vi "TestSequenceSubVI.vi"(0 "GuiRef":T2={"StringOut"=refnum, "AbortOnFail"=refnum, "SN"=refnum, "SN_Length"=refnum, "TestResult"=refnum, "CycleTime"=refnum, "ErrorCode"=refnum, "UUTStatus"=refnum, "DataBaseEnable?"=refnum, "DUTModel"=refnum, "FixtureID"=refnum, "OperatorID"=refnum, "SNReady"=refnum, "StopSlot"=refnum, "NextStep"=refnum, "PassYeild"=refnum, "Failed"=refnum, "Passed"=refnum, "Tested"=refnum, "TestItemsCtl"={"StepName"="", "TestEnable"=FALSE, "LoopCount"=0, "StopOnFail"=FALSE, "Index"=0, "TestName"="", "通道"="", "参数"="", "TimeStart"=0}, "ProcessBar"=refnum, "Slot"=enum."Slot1", "Row"=3, "States"=refnum, "TestMode"=refnum, "循环次数-DUT"=refnum, "波形图"=refnum, "产品型号"=refnum, "子面板"=refnum, "测试失败项目"=refnum, "测试结果"=refnum, "DUT"=refnum, "Starttime"=refnum, "SlotReady"=refnum, "版本信息"=refnum}, 7 "MSComm":refnum<k7>, 11 "error in":errorcluster, 14 "semaphore":T1 caption="信号量") -> (15 "error out":errorcluster)   [LabVIEW 2013]
uses:
  SystemCode/SysControl/Reference.ctl
  SystemCode/SysControl/TestItemsCTL.ctl
  SystemCode/SysControl/Slot.ctl
  SourceCode/CCID info.ctl
  <vilib>/measure/matone.llb/Extract Single Tone Information 1 Chan.vi
  SourceCode/GlobalValue.vi
  <vilib>/measure/madcrms.llb/Basic Averaged DC-RMS for 1 Chan.vi
  <vilib>/measure/matone.llb/SINAD Analyzer 1 Chan.vi
  <vilib>/addons/Sound and Vibration/svt_Distortion/SVT THD+N (Time) (1 Ch).vi
  <vilib>/ErrorRing/Error Ring.xnode
  <vilib>/measure/NI_MAPro.lvlib
  <vilib>/addons/Sound and Vibration/svt_Distortion/SoundVib_Distortion.lvlib
panel:
  out "错误输出":errorcluster
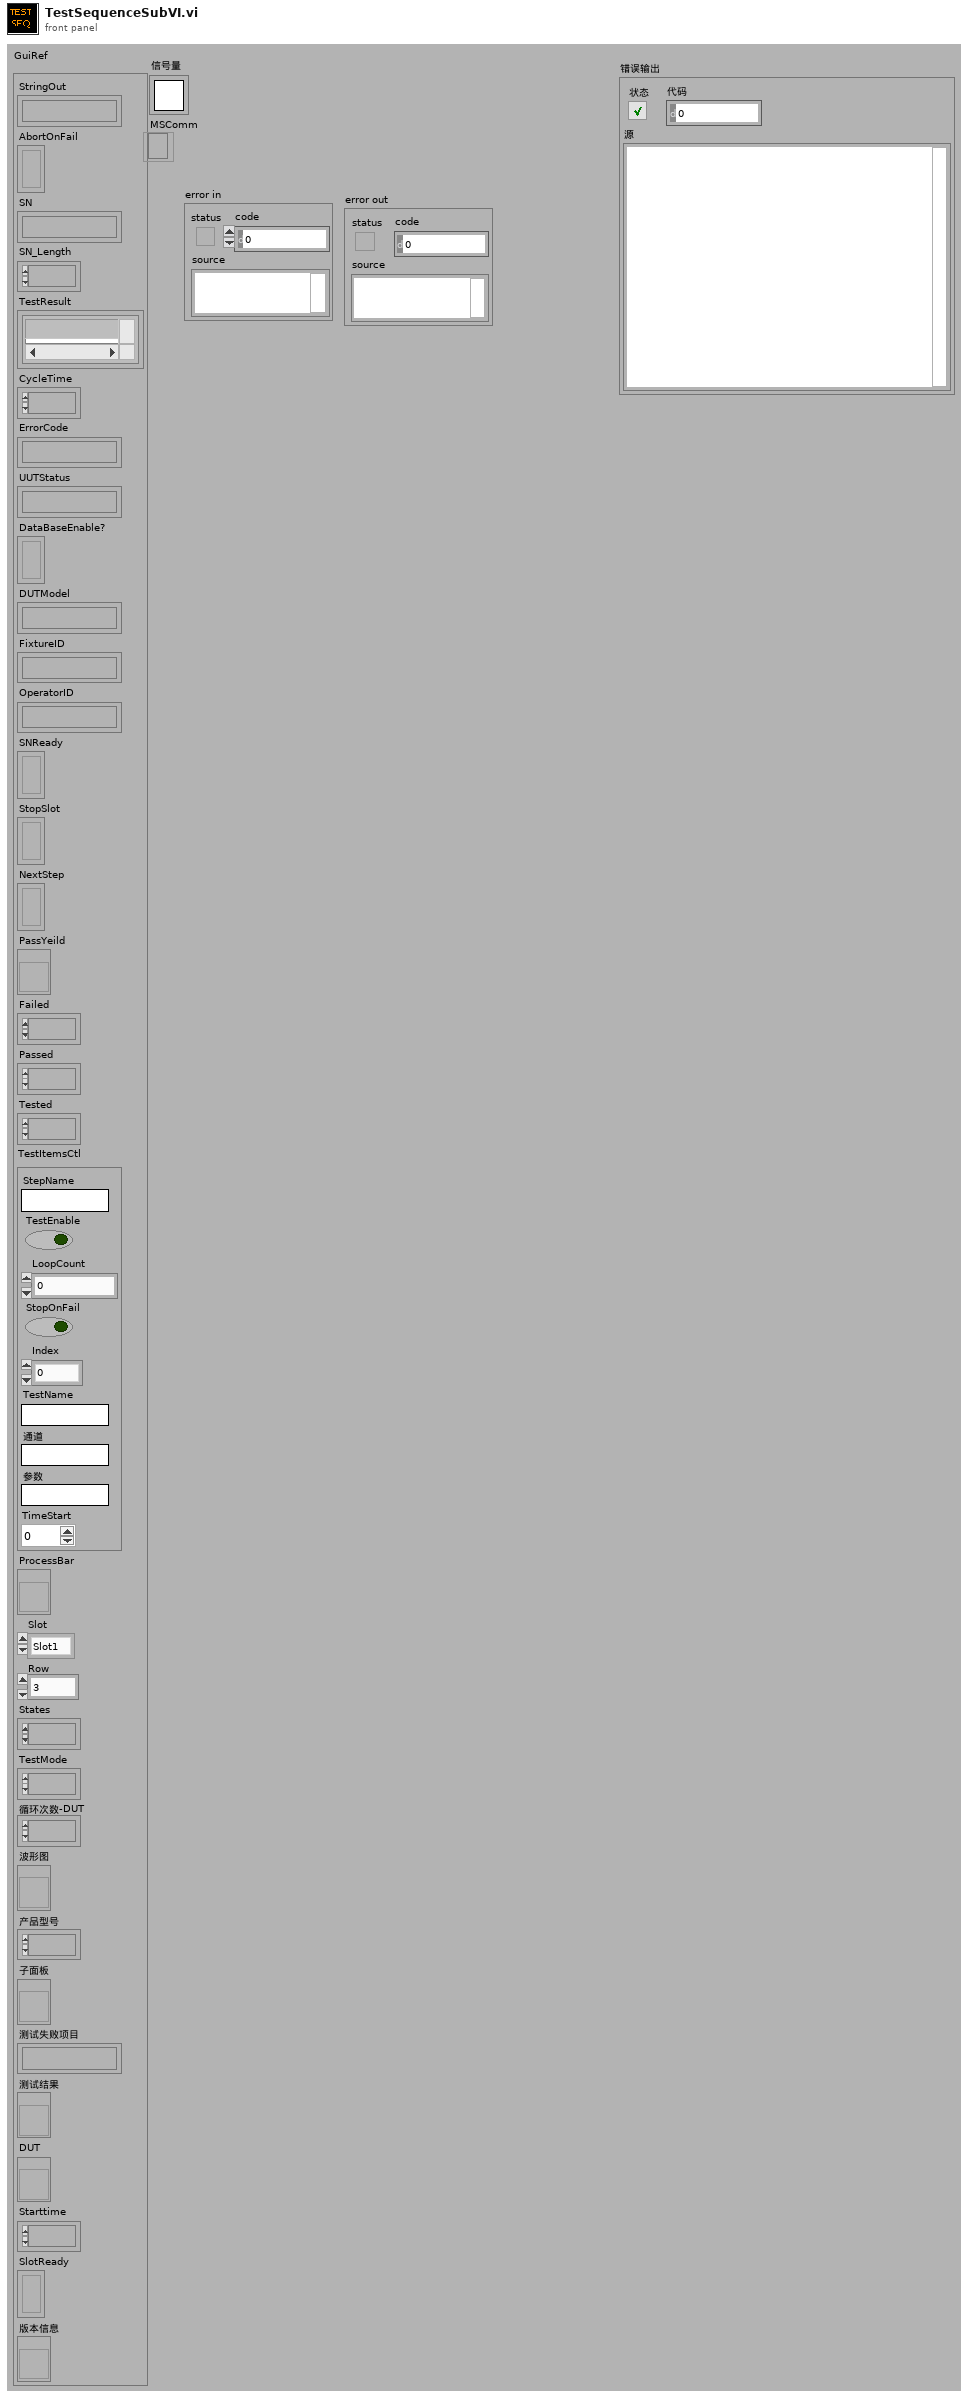
[diagram p1: front panel]
types:
  T1 = typedef "Semaphore RefNum" = refnum<k1>
  T2 = typedef "Reference.ctl" = cluster{"StringOut":refnum<vi>, "AbortOnFail":refnum<vi>, "SN":refnum<vi>, "SN_Length":refnum<vi>, "TestResult":refnum<vi>, "CycleTime":refnum<vi>, "ErrorCode":refnum<vi>, "UUTStatus":refnum<vi>, "DataBaseEnable?":refnum<vi>, "DUTModel":refnum<vi>, "FixtureID":refnum<vi>, "OperatorID":refnum<vi>, "SNReady":refnum<vi>, "StopSlot":refnum<vi>, "NextStep":refnum<vi>, "PassYeild":refnum<vi>, "Failed":refnum<vi>, "Passed":refnum<vi>, "Tested":refnum<vi>, "TestItemsCtl":T3, "ProcessBar":refnum<vi>, "Slot":T4, "Row":u32, "States":refnum<vi>, "TestMode":refnum<vi>, "循环次数-DUT":refnum<vi>, "波形图":refnum<vi>, "产品型号":refnum<vi>, "子面板":refnum<vi>, "测试失败项目":refnum<vi>, "测试结果":refnum<vi>, "DUT":refnum<vi>, "Starttime":refnum<vi>, "SlotReady":refnum<vi>, "版本信息":refnum<vi>}
  T3 = typedef "TestItemsCTL.ctl" = cluster{"StepName":string, "TestEnable":bool, "LoopCount":i32, "StopOnFail":bool, "Index":u32, "TestName":string, "通道":string, "参数":string, "TimeStart":u32}
  T4 = typedef "Slot.ctl" = enum16{"Slot1", "Slot2", "Slot3", "Slot4"}
  T5 = cluster{"THD+N units":enum16{"dB", "linear ratio", "%"}, "detected fundamental amplitude units":enum16{"EU rms", "EU peak", "EU peak-peak"}}
  T6 = typedef "CCID info.ctl" = enum16{"Fw Ver", "HW Ver", "CCID", "WiFiName", "DevID"}
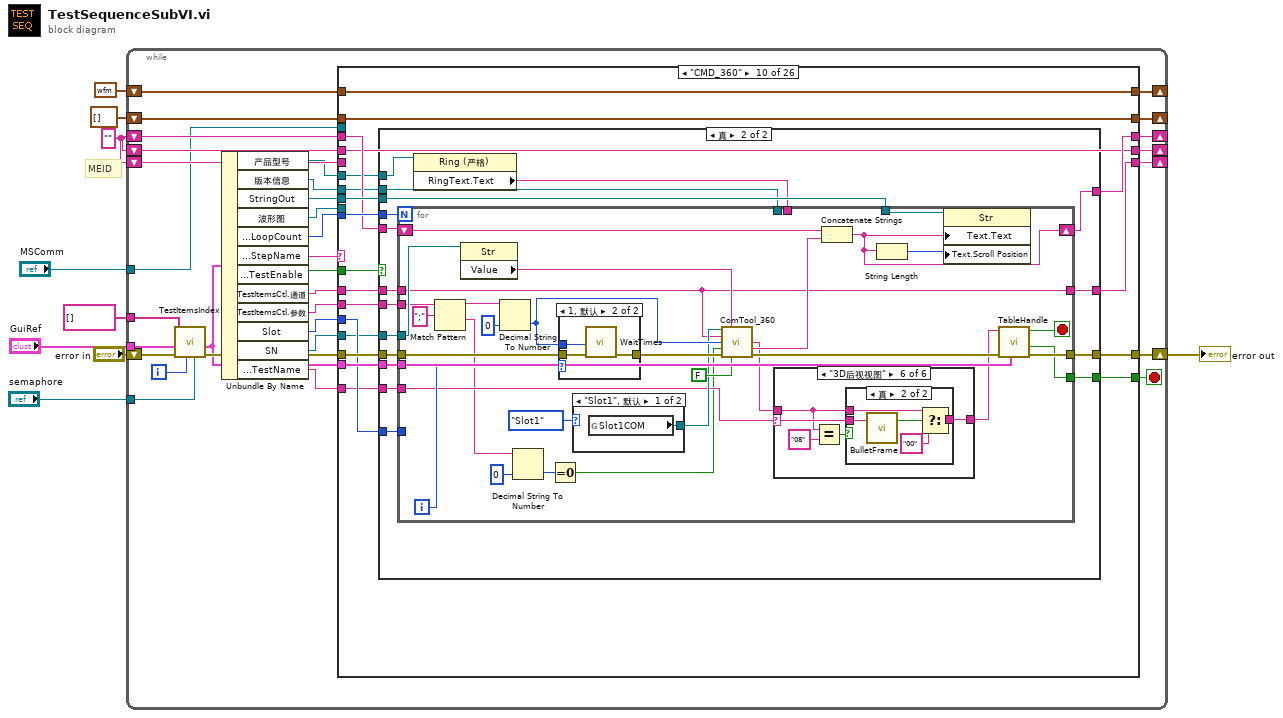
[diagram p0: block diagram]
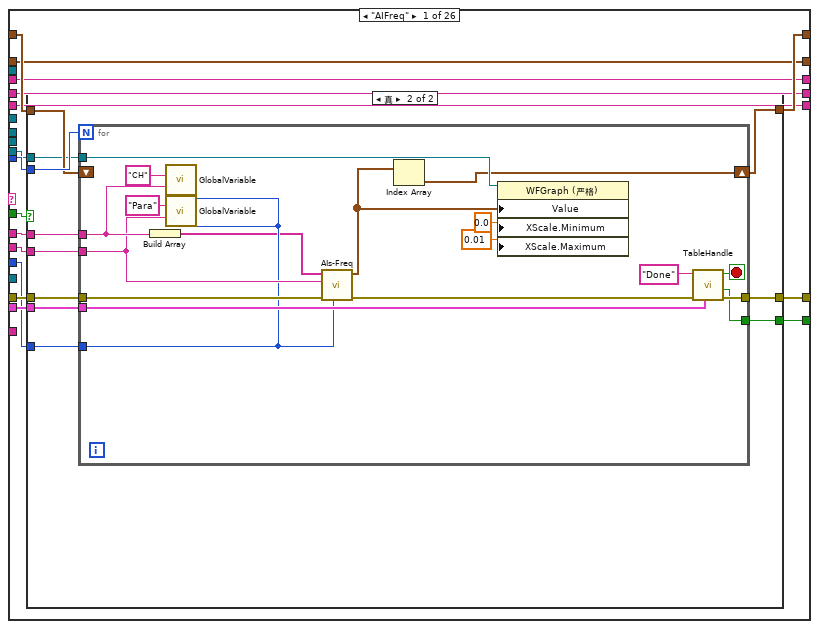
[diagram p2: hidden frame]
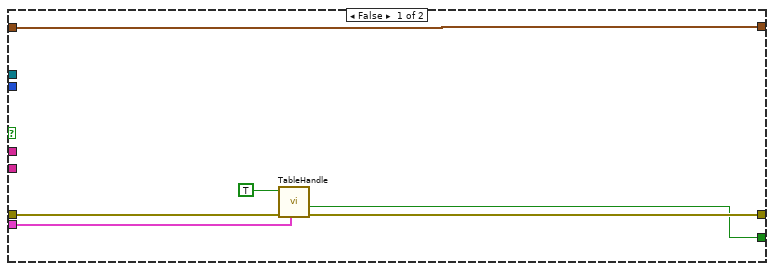
[diagram p3: hidden frame]
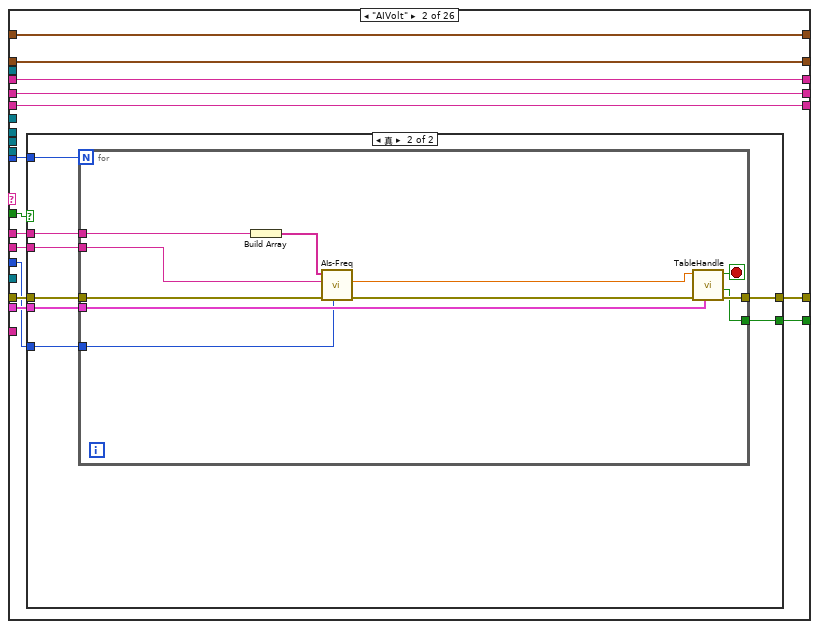
[diagram p4: hidden frame]
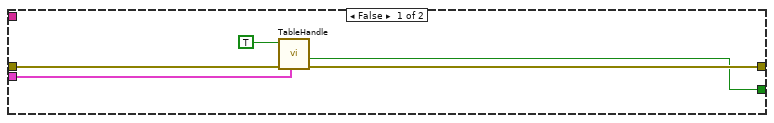
[diagram p5: hidden frame]
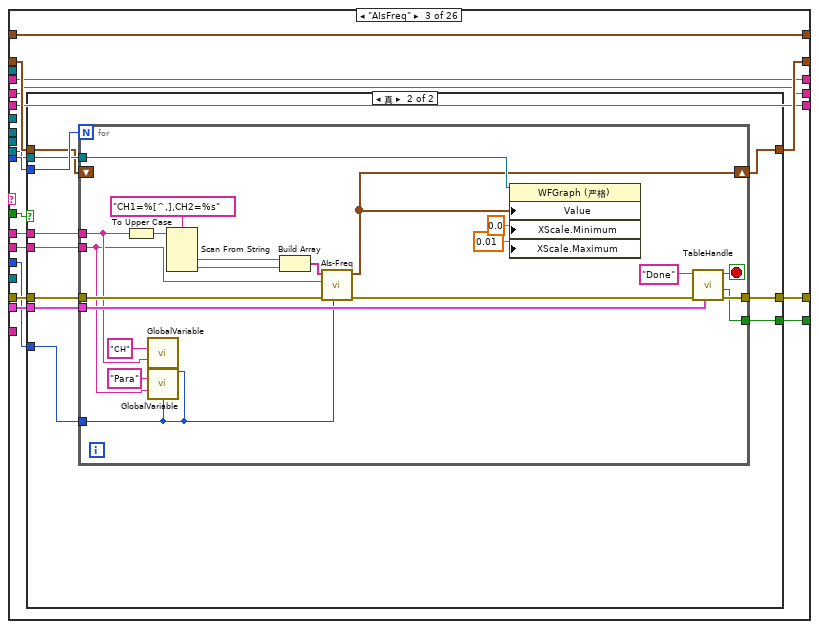
[diagram p6: hidden frame]
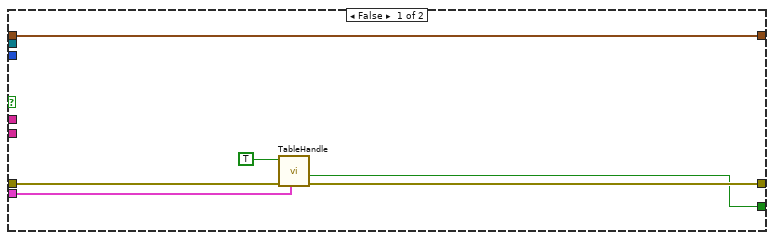
[diagram p7: hidden frame]
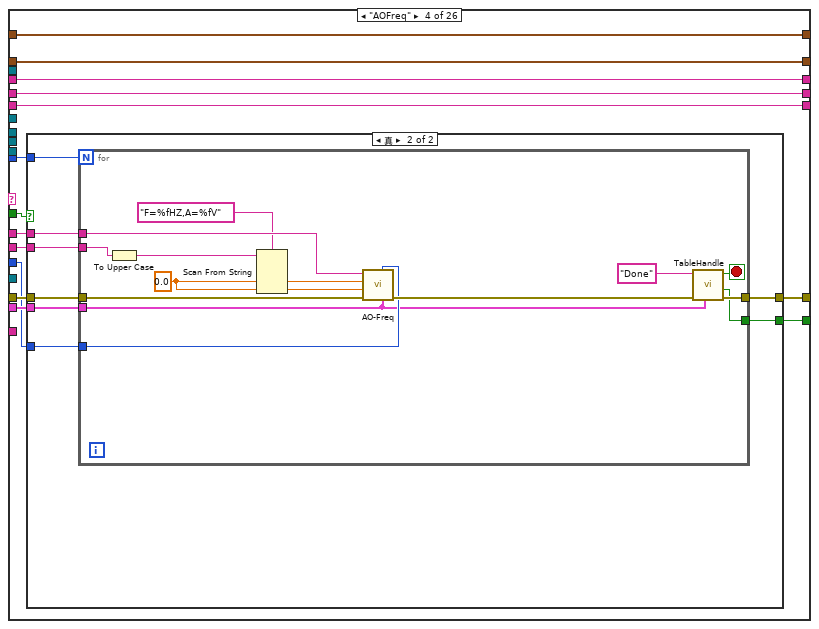
[diagram p8: hidden frame]
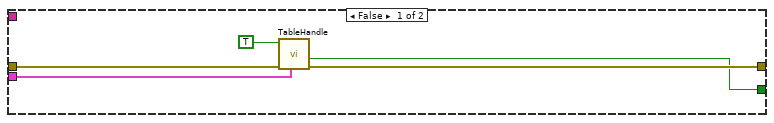
[diagram p9: hidden frame]
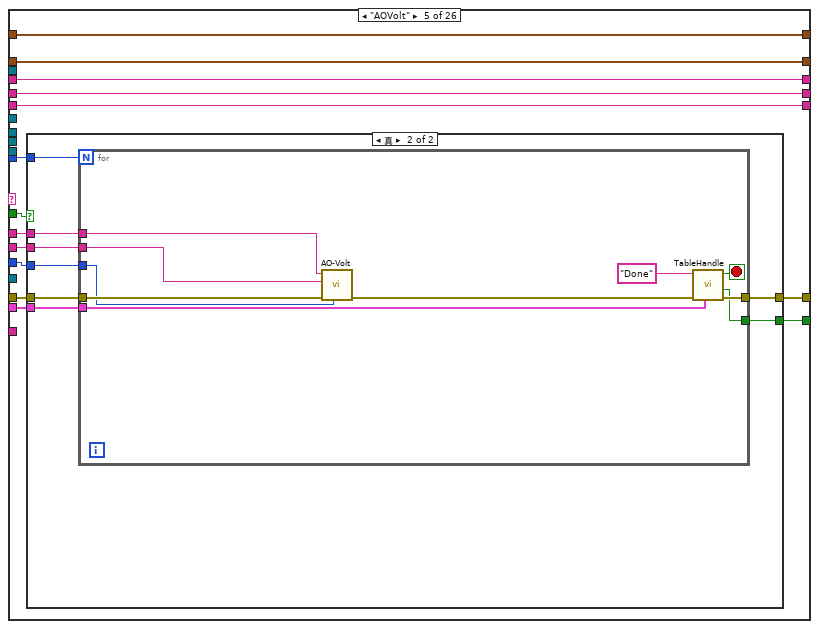
[diagram p10: hidden frame]
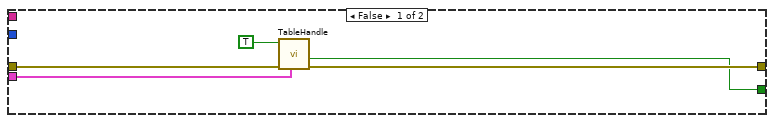
[diagram p11: hidden frame]
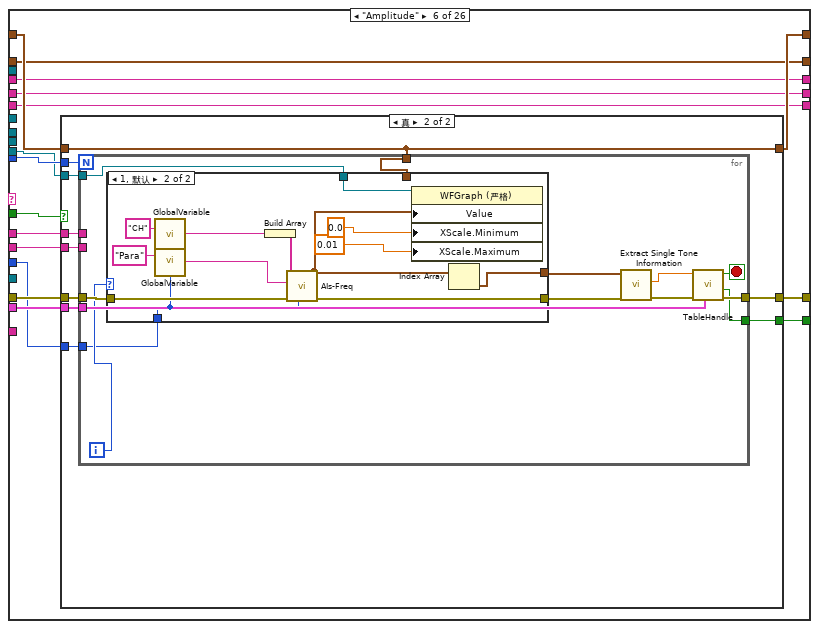
[diagram p12: hidden frame]
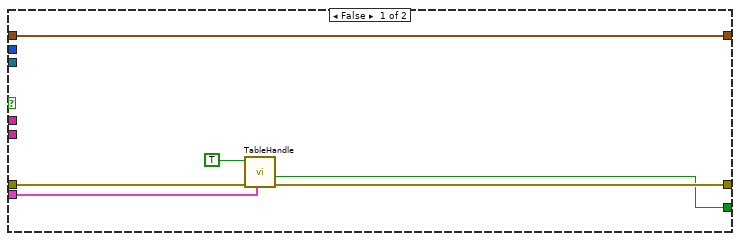
[diagram p13: hidden frame]
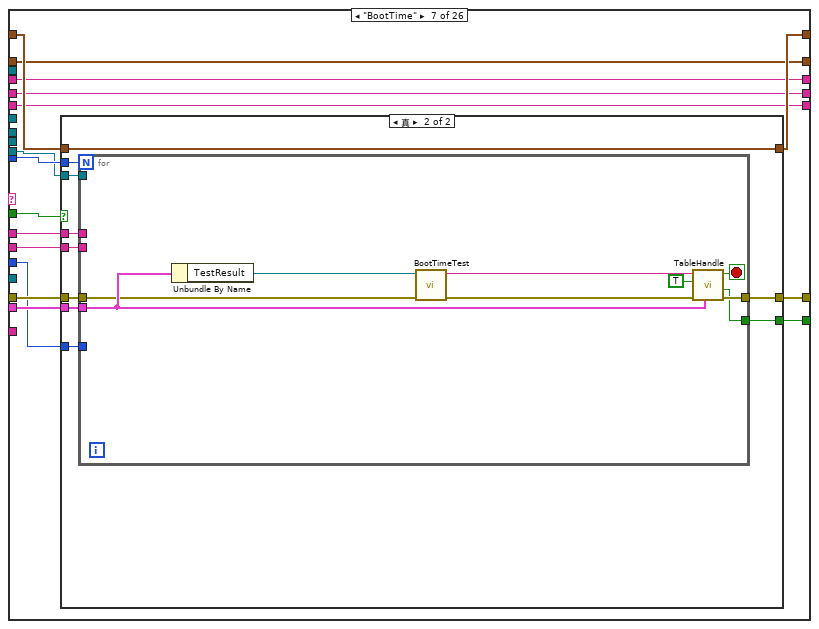
[diagram p15: hidden frame]
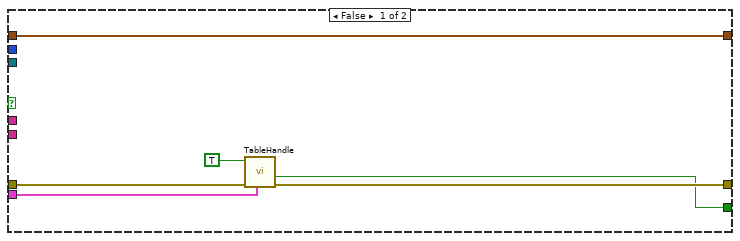
[diagram p16: hidden frame]
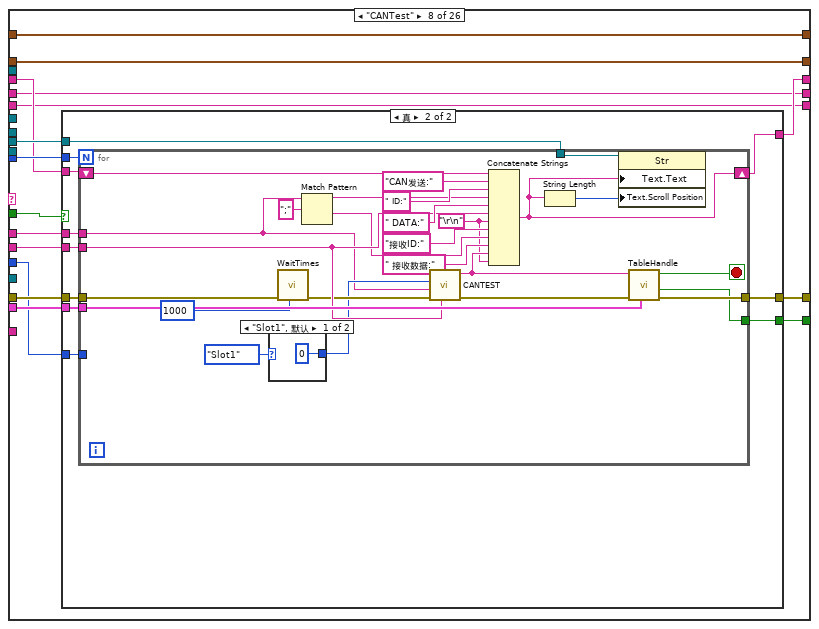
[diagram p17: hidden frame]
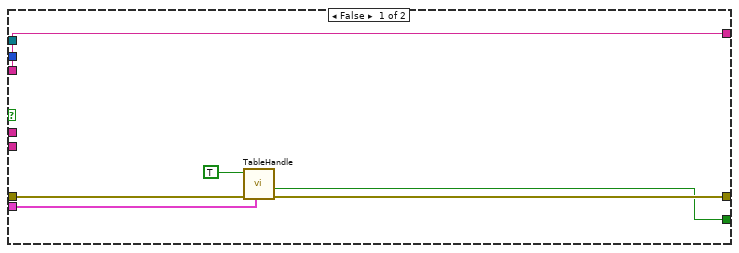
[diagram p18: hidden frame]
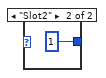
[diagram p19: hidden frame]
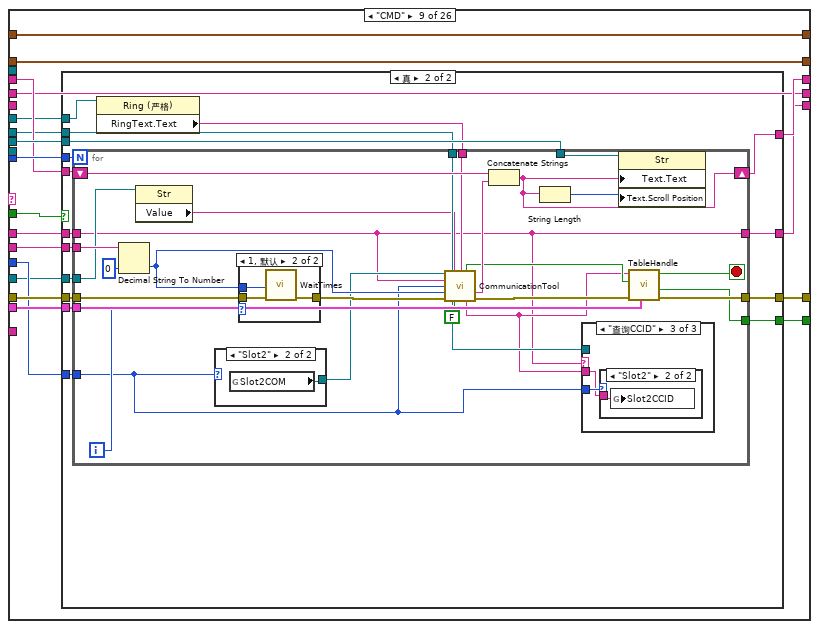
[diagram p20: hidden frame]
diagram:
  w2 = "" ("CMD")
  # "MEID"
  n1 = while {
    shift-right: [w37] -> w9
    shift-left: "error in" -> [w41]
    tunnel: "GuiRef" -> [w35]
    shift-right: [w29] -> _
    shift-left: waveform(dbl) {"t0"=timestamp(0 s since 1904-01-01), "dt"=1.0, "Y"=[]} ("Raw Data 3") -> [w28]
    shift-right: [w27] -> _
    shift-left: waveform(dbl)[] [] ("波形图") -> [w26]
    shift-right: [w23] -> _
    shift-left: w2 -> [w22]
    tunnel: string[] [] ("Fail项目") -> [w21]
    tunnel: "semaphore" -> [w19]
    shift-right: [w18] -> _
    shift-left: w2 -> [w17]
    shift-right: [w15] -> _
    shift-left: w2 -> [w16]
    tunnel: "MSComm" -> [w11]
    i -> [w20]
    stop <- w36 stop-if-true
    n2 = call "TestItemsIndex.vi"("semaphore"=w19, "TestItemIndexIn"=w20, "ErrorIn(NoError)"=w41, "GuiRef"=w35, "Fail项目"=w21) -> ("ErrorOut"=w40:errorcluster, "GuiRefOut"=w34:T2)  [unwired: 5 out]
    n3 = Unbundle By Name(w34) -> ("产品型号"=w12:refnum<vi>, "版本信息"=w14:refnum<vi>, "StringOut"=w24:refnum<vi>, "波形图"=w25:refnum<vi>, "TestItemsCtl.LoopCount"=w30:i32, "TestItemsCtl.StepName"=w39:string, "TestItemsCtl.TestEnable"=w38:bool, "TestItemsCtl.通道"=w31:string, "TestItemsCtl.参数"=w32:string, "Slot"=w33:T4, "SN"=w13:refnum<vi>, "TestItemsCtl.TestName"=w10:string)
    n4 = case shown="\"CMD_360\"" w39 {
      selector: w39 -> [_ _ _ _ _ _ _ _ _ _ _ _ _ _ _ _ _ _ _ _ _ _ _ _ _ w1271]
      tunnel: [w55 w104 w144 w196 w238 w277 w337 w378 w442 w522 w654 w694 w730 w767 w807 w844 w907 w967 w1035 w1063 w1117 w1131 w1187 w1223 w1236 w1275] -> w37
      tunnel: w40 -> [w56 w105 w145 w197 w239 w278 w338 w379 w443 w523 w655 w695 w731 w768 w808 w845 w908 w968 w1036 w1067 w1117 w1132 _ w1223 w1237 _]
      tunnel: w34 -> [w57 w106 w146 w198 w240 w279 w339 w380 w444 w524 w656 w696 w732 w769 w809 w846 w909 w969 w1037 w1066 _ w1133 w1182 _ w1238 _]
      tunnel: w38 -> [w54 w103 w143 w195 w237 w276 w336 w377 w441 w521 w653 w693 w729 w766 w806 w843 w906 w966 w1034 w1061 _ w1130 _ _ w1235 _]
      tunnel: [w53 w102 w142 w194 w236 w275 w335 w376 w440 w520 w652 w692 w728 w765 w805 w842 w905 w965 w1033 w1064 TRUE ("StopOnFail?") w1129 w1186 FALSE ("StopOnFail?") w1234 TRUE ("StopOnFail?")] -> w36
      tunnel: w33 -> [w52 w101 w141 w193 w235 w274 w334 w375 w439 w519 w651 w691 w727 w764 w804 w841 w904 w964 w1032 w1065 _ w1128 w1190 _ w1233 w1266]
      tunnel: w32 -> [w50 w99 w139 w191 w233 w272 w332 w373 w437 w517 w649 w689 w725 w762 w802 w839 w902 w962 w1030 w1068 _ w1126 _ _ w1231 _]
      tunnel: w31 -> [w51 w100 w140 w192 w234 w273 w333 w374 w438 w518 w650 w690 w726 w763 w803 w840 w903 w963 w1031 w1069 _ w1127 w1191 _ w1232 _]
      tunnel: w30 -> [w49 w98 w138 w190 w232 w271 w331 w372 w436 w516 w648 w688 w724 w761 w801 w838 w901 w961 w1029 w1070 _ w1125 _ _ w1230 _]
      tunnel: [w48 w97 w137 w189 w231 w269 w329 w371 w435 w515 w646 w687 w723 w760 w799 w837 w899 w959 w1028 w1062 w1115 w1123 w1184 w1221 w1228 w1274] -> w29
      tunnel: w28 -> [w47 w97 w137 w189 w231 w270 w330 w371 w435 w515 w647 w687 w723 w760 w800 w837 w900 w960 w1028 w1062 w1115 w1124 w1184 w1221 w1229 w1274]
      tunnel: [w46 w96 w136 w188 w230 w268 w328 w370 w434 w514 w645 w686 w722 w759 w798 w836 w898 w958 w1027 w1074 w1114 w1122 w1195 w1220 w1227 w1273] -> w27
      tunnel: w26 -> [w46 w96 w135 w188 w230 w268 w328 w370 w434 w514 w645 w686 w722 w759 w798 w836 w898 w958 w1027 w1074 w1114 w1122 w1195 w1220 w1227 w1273]
      tunnel: w25 -> [w45 _ w134 _ _ w266 w326 _ _ _ _ _ _ _ _ _ w896 w956 _ _ _ w1120 _ _ _ _]
      tunnel: w24 -> [_ _ _ _ _ _ _ w369 w433 w513 _ _ _ _ _ _ _ _ _ _ _ _ _ _ _ _]
      tunnel: [w44 w95 w133 w187 w229 w267 w327 w368 w432 w512 w644 w685 w721 w758 w797 w835 w897 w957 w1026 w1073 w1113 w1121 w1194 w1219 w1226 w1268] -> w23
      tunnel: w22 -> [w44 w95 w133 w187 w229 w267 w327 w367 w431 w511 w644 w685 w721 w758 w797 w835 w897 w957 w1026 w1073 w1113 w1121 w1194 w1219 w1226 w1268]
      tunnel: [w43 w94 w132 w186 w228 w265 w325 w366 w430 w510 w643 w684 w720 w757 w796 w834 w895 w955 w1025 w1072 w1112 w1119 w1193 w1218 w1225 w1264] -> w18
      tunnel: w17 -> [w43 w94 w132 w186 w228 w265 w325 w366 w430 w510 w643 w684 w720 w757 w796 w834 w895 w955 w1025 w1072 w1112 w1119 w1193 w1218 w1225 w1264]
      tunnel: w16 -> [w42 w93 w131 w185 w227 w264 w324 w365 _ _ w642 w683 w719 w756 w795 w833 w894 w954 w1024 w1071 w1111 w1118 w1192 w1217 w1224 w1263]
      tunnel: [w42 w93 w131 w185 w227 w264 w324 w365 w429 w509 w642 w683 w719 w756 w795 w833 w894 w954 w1024 w1071 w1111 w1118 w1192 w1217 w1224 w1263] -> w15
      tunnel: w14 -> [_ _ _ _ _ _ _ _ w428 w508 _ _ _ _ _ _ _ _ _ _ _ _ _ _ _ _]
      tunnel: w13 -> [_ _ _ _ _ _ _ _ w427 w507 w641 _ _ _ _ _ _ _ _ _ _ _ w1188 _ _ _]
      tunnel: w12 -> [_ _ _ _ _ _ _ _ w426 w506 _ _ _ _ _ _ _ _ _ _ _ _ w1189 _ _ _]
      tunnel: w11 -> [_ _ _ _ _ _ _ _ _ _ _ _ _ _ _ _ _ _ _ _ _ _ _ _ _ _]
      tunnel: w10 -> [_ _ _ _ _ _ _ _ _ w505 _ _ _ _ _ _ _ _ _ _ _ _ _ _ _ _]
      frame "AIFreq" {
        n5 = case shown="真" w54 {
          tunnel: w57 -> [w61 w72]
          tunnel: w56 -> [w62 w74]
          tunnel: [w63 w73] -> w55
          tunnel: [w60 w71] -> w53
          tunnel: w52 -> [_ w70]
          tunnel: w51 -> [_ w69]
          tunnel: w50 -> [_ w68]
          tunnel: w49 -> [_ w67]
          tunnel: [w58 w66] -> w48
          tunnel: w47 -> [w58 w65]
          tunnel: w45 -> [_ w64]
          frame False {
            n6 = call "TableHandle.vi"("All"=w61, "error in (no error)"=w62, "DataIn"=TRUE) -> ("error out"=w63:errorcluster, "Stop?"=w60:bool)  [unwired: 3 in, 4 out]
          }
          frame True {
            n7 = for "For循环" {
              N: w67 -> [_]
              tunnel: w74 -> [w88]
              tunnel: [w92] -> w73
              tunnel: w72 -> [w89]
              tunnel: [w90] -> w71
              tunnel: w70 -> [w77]
              tunnel: w68 -> [w78]
              tunnel: w69 -> [w80]
              shift-right: [w82] -> w66
              shift-left: w65 -> [_]
              tunnel: w64 -> [w84]
              stop <- w91 stop-if-true
              n8 = Build Array(w80) -> (w76:string[])
              n9 = call "GlobalVariable.vi"("Name"="CH", "ValueIn"=w80, "Slot"=w77) -> ()  [unwired: 9 in, 4 out]
              n10 = call "GlobalVariable.vi"("Name"="Para", "ValueIn"=w78, "Slot"=w77) -> ()  [unwired: 9 in, 4 out]
              n11 = call "AIs-Freq.vi"("Slot"=w77, "error in"=w88, "Mode"=w78, "CHs"=w76) -> ("error out"=w87:errorcluster, "波形图"=w75:waveform(dbl)[])  [unwired: 5 in, 1 out]
              n12 = Index Array(array=w75) -> (element=w82:waveform(dbl))  [unwired: 1 in]
              n13 = property class="WFGraph (严格)"(reference=w84, "Value"=w75, "XScale.Minimum"=0.0 ("X标尺.范围:最小值"), "XScale.Maximum"=0.01 ("X标尺.范围:最大值")) -> ()  [unwired: 1 in, 2 out]
              n14 = call "TableHandle.vi"("All"=w89, "error in (no error)"=w87, "DataIn"="Done") -> ("error out"=w92:errorcluster, "Stop?"=w90:bool, "StopForLoop"=w91:bool)  [unwired: 4 in, 2 out]
            }
          }
        }
      }
      frame "AIVolt" {
        n15 = case shown="真" w103 {
          tunnel: w106 -> [w109 w117]
          tunnel: w105 -> [w110 w119]
          tunnel: [w111 w118] -> w104
          tunnel: [w108 w116] -> w102
          tunnel: w101 -> [_ w115]
          tunnel: w100 -> [_ w114]
          tunnel: w99 -> [_ w113]
          tunnel: w98 -> [_ w112]
          frame False {
            n16 = call "TableHandle.vi"("All"=w109, "error in (no error)"=w110, "DataIn"=TRUE) -> ("error out"=w111:errorcluster, "Stop?"=w108:bool)  [unwired: 3 in, 4 out]
          }
          frame True {
            n17 = for "For循环" {
              N: w112 -> [_]
              tunnel: w119 -> [w126]
              tunnel: [w130] -> w118
              tunnel: w117 -> [w127]
              tunnel: [w128] -> w116
              tunnel: w115 -> [w123]
              tunnel: w113 -> [w124]
              tunnel: w114 -> [w122]
              stop <- w129 stop-if-true
              n18 = Build Array(w122) -> (w121:string[])
              n19 = call "AIs-Freq.vi"("Slot"=w123, "error in"=w126, "Mode"=w124, "CHs"=w121) -> ("error out"=w125:errorcluster, "RMS value"=w120:dbl)  [unwired: 5 in, 1 out]
              n20 = call "TableHandle.vi"("All"=w127, "error in (no error)"=w125, "DataIn"=w120) -> ("error out"=w130:errorcluster, "Stop?"=w128:bool, "StopForLoop"=w129:bool)  [unwired: 4 in, 2 out]
            }
          }
        }
      }
      frame "AIsFreq" {
        n21 = case shown="真" w143 {
          tunnel: w146 -> [w150 w161]
          tunnel: w145 -> [w151 w163]
          tunnel: [w152 w162] -> w144
          tunnel: [w149 w160] -> w142
          tunnel: w141 -> [_ w159]
          tunnel: w140 -> [_ w158]
          tunnel: w139 -> [_ w157]
          tunnel: w138 -> [_ w156]
          tunnel: [w147 w155] -> w136
          tunnel: w135 -> [w147 w153]
          tunnel: w134 -> [_ w154]
          frame False {
            n22 = call "TableHandle.vi"("All"=w150, "error in (no error)"=w151, "DataIn"=TRUE) -> ("error out"=w152:errorcluster, "Stop?"=w149:bool)  [unwired: 3 in, 4 out]
          }
          frame True {
            n23 = for "For循环" {
              N: w156 -> [_]
              tunnel: w163 -> [w180]
              tunnel: [w184] -> w162
              tunnel: w161 -> [w181]
              tunnel: [w182] -> w160
              tunnel: w159 -> [w166]
              tunnel: w157 -> [w167]
              tunnel: w158 -> [w168]
              shift-right: [w164] -> w155
              shift-left: w153 -> [_]
              tunnel: w154 -> [w173]
              stop <- w183 stop-if-true
              n24 = To Upper Case(1:w168) -> (0:w177:string)
              n25 = call "GlobalVariable.vi"("Name"="CH", "ValueIn"=w168, "Slot"=w166) -> ()  [unwired: 9 in, 4 out]
              n26 = call "GlobalVariable.vi"("Name"="Para", "ValueIn"=w167, "Slot"=w166) -> ()  [unwired: 9 in, 4 out]
              n27 = Scan From String(format string="CH1=%[^,],CH2=%s" ("格式字符串"), input string=w177) -> (output 1=w175:string, output 2=w174:string)  [unwired: 4 in, 3 out]
              n28 = Build Array(w175, w174) -> (w165:string[])
              n29 = call "AIs-Freq.vi"("Slot"=w166, "error in"=w180, "Mode"=w167, "CHs"=w165) -> ("error out"=w179:errorcluster, "波形图"=w164:waveform(dbl)[])  [unwired: 5 in, 1 out]
              n30 = property class="WFGraph (严格)"(reference=w173, "Value"=w164, "XScale.Minimum"=0.0 ("X标尺.范围:最小值"), "XScale.Maximum"=0.01 ("X标尺.范围:最大值")) -> ()  [unwired: 1 in, 2 out]
              n31 = call "TableHandle.vi"("All"=w181, "error in (no error)"=w179, "DataIn"="Done") -> ("error out"=w184:errorcluster, "Stop?"=w182:bool, "StopForLoop"=w183:bool)  [unwired: 4 in, 2 out]
            }
          }
        }
      }
      frame "AOFreq" {
        n32 = case shown="真" w195 {
          tunnel: w198 -> [w201 w209]
          tunnel: w197 -> [w202 w211]
          tunnel: [w203 w210] -> w196
          tunnel: [w200 w208] -> w194
          tunnel: w193 -> [_ w207]
          tunnel: w192 -> [_ w206]
          tunnel: w191 -> [_ w205]
          tunnel: w190 -> [_ w204]
          frame False {
            n33 = call "TableHandle.vi"("All"=w201, "error in (no error)"=w202, "DataIn"=TRUE) -> ("error out"=w203:errorcluster, "Stop?"=w200:bool)  [unwired: 3 in, 4 out]
          }
          frame True {
            n34 = for "For循环" {
              N: w204 -> [_]
              tunnel: w211 -> [w223]
              tunnel: [w226] -> w210
              tunnel: w209 -> [w212]
              tunnel: [w224] -> w208
              tunnel: w207 -> [w213]
              tunnel: w205 -> [w218]
              tunnel: w206 -> [w221]
              stop <- w225 stop-if-true
              w217 = 0.0 ("默认值 1")
              n35 = To Upper Case(1:w218) -> (0:w216:string)
              n36 = Scan From String(format string="F=%fHZ,A=%fV" ("格式字符串"), input string=w216, default 1=w217, default 2=w217) -> (output 1=w215:dbl, output 2=w214:dbl)  [unwired: 2 in, 3 out]
              n37 = call "AO-Freq.vi"("GuiRef"=w212, "Slot"=w213, "error in"=w223, "AMP"=w214, "Freq"=w215, "CH"=w221) -> ("error out"=w222:errorcluster)  [unwired: 5 in]
              n38 = call "TableHandle.vi"("All"=w212, "error in (no error)"=w222, "DataIn"="Done") -> ("error out"=w226:errorcluster, "Stop?"=w224:bool, "StopForLoop"=w225:bool)  [unwired: 4 in, 2 out]
            }
          }
        }
      }
      frame "AOVolt" {
        n39 = case shown="真" w237 {
          tunnel: w240 -> [w243 w251]
          tunnel: w239 -> [w244 w253]
          tunnel: [w245 w252] -> w238
          tunnel: [w242 w250] -> w236
          tunnel: w235 -> [_ w249]
          tunnel: w234 -> [_ w248]
          tunnel: w233 -> [_ w247]
          tunnel: w232 -> [_ w246]
          frame False {
            n40 = call "TableHandle.vi"("All"=w243, "error in (no error)"=w244, "DataIn"=TRUE) -> ("error out"=w245:errorcluster, "Stop?"=w242:bool)  [unwired: 3 in, 4 out]
          }
          frame True {
            n41 = for "For循环" {
              N: w246 -> [_]
              tunnel: w253 -> [w259]
              tunnel: [w263] -> w252
              tunnel: w251 -> [w260]
              tunnel: [w261] -> w250
              tunnel: w249 -> [w254]
              tunnel: w247 -> [w255]
              tunnel: w248 -> [w257]
              stop <- w262 stop-if-true
              n42 = call "AO-Volt.vi"("Slot"=w254, "error in"=w259, "Value"=w255, "CH"=w257) -> ("error out"=w258:errorcluster)  [unwired: 7 in]
              n43 = call "TableHandle.vi"("All"=w260, "error in (no error)"=w258, "DataIn"="Done") -> ("error out"=w263:errorcluster, "Stop?"=w261:bool, "StopForLoop"=w262:bool)  [unwired: 4 in, 2 out]
            }
          }
        }
      }
      frame "Amplitude" {
        n44 = case shown="真" w276 {
          tunnel: w279 -> [w283 w293]
          tunnel: w278 -> [w284 w295]
          tunnel: [w285 w294] -> w277
          tunnel: [w282 w292] -> w275
          tunnel: w274 -> [_ w291]
          tunnel: w273 -> [_ w290]
          tunnel: w272 -> [_ w289]
          tunnel: w271 -> [_ w288]
          tunnel: w270 -> [w280 w287]
          tunnel: [w280 w287] -> w269
          tunnel: w266 -> [_ w286]
          frame False {
            n45 = call "TableHandle.vi"("All"=w283, "error in (no error)"=w284, "DataIn"=TRUE) -> ("error out"=w285:errorcluster, "Stop?"=w282:bool)  [unwired: 3 in, 4 out]
          }
          frame True {
            n46 = for "For循环" {
              N: w288 -> [_]
              tunnel: w295 -> [w302]
              tunnel: [w308] -> w294
              tunnel: w293 -> [w305]
              tunnel: [w306] -> w292
              tunnel: w291 -> [w296]
              tunnel: w289 -> [_]
              tunnel: w290 -> [_]
              tunnel: w287 -> [w299]
              tunnel: w286 -> [w297]
              i -> [w300]
              stop <- w307 stop-if-true
              n47 = case shown="1, 默认" w300 {
                tunnel: w302 -> [w310 w321]
                tunnel: [w310 w320] -> w301
                tunnel: w297 -> [_ w319]
                tunnel: w296 -> [_ w315]
                tunnel: [w309 w316] -> w298
                tunnel: w299 -> [w309 _]
                frame 0 {
                }
                frame 1, Default {
                  n48 = call "GlobalVariable.vi"("Name"="CH", "Slot"=w315) -> ("String"=w314:string)  [unwired: 10 in, 3 out]
                  n49 = call "GlobalVariable.vi"("Name"="Para", "Slot"=w315) -> ("String"=w313:string)  [unwired: 10 in, 3 out]
                  n50 = Build Array(w314) -> (w318:string[])
                  n51 = call "AIs-Freq.vi"("Slot"=w315, "error in"=w321, "Mode"=w313, "CHs"=w318) -> ("error out"=w320:errorcluster, "波形图"=w317:waveform(dbl)[])  [unwired: 5 in, 1 out]
                  n52 = property class="WFGraph (严格)"(reference=w319, "Value"=w317, "XScale.Minimum"=0.0 ("X标尺.范围:最小值"), "XScale.Maximum"=0.01 ("X标尺.范围:最大值")) -> ()  [unwired: 1 in, 2 out]
                  n53 = Index Array(array=w317) -> (element=w316:waveform(dbl))  [unwired: 1 in]
                }
              }
              n54 = call-poly <vilib>:"Extract Single Tone Information.vi"("error in (no error)"=w301, "time signal in"=w298) -> ("error out"=w304:errorcluster, "detected amplitude"=w303:dbl)  [unwired: 4 in, 4 out]
              n55 = call "TableHandle.vi"("All"=w305, "error in (no error)"=w304, "DataIn"=w303) -> ("error out"=w308:errorcluster, "Stop?"=w306:bool, "StopForLoop"=w307:bool)  [unwired: 4 in, 2 out]
            }
          }
        }
      }
      frame "BootTime" {
        n56 = case shown="真" w336 {
          tunnel: w339 -> [w343 w353]
          tunnel: w338 -> [w344 w355]
          tunnel: [w345 w354] -> w337
          tunnel: [w342 w352] -> w335
          tunnel: w334 -> [_ w351]
          tunnel: w333 -> [_ w350]
          tunnel: w332 -> [_ w349]
          tunnel: w331 -> [_ w348]
          tunnel: w330 -> [w340 w346]
          tunnel: [w340 w346] -> w329
          tunnel: w326 -> [_ w347]
          frame False {
            n57 = call "TableHandle.vi"("All"=w343, "error in (no error)"=w344, "DataIn"=TRUE) -> ("error out"=w345:errorcluster, "Stop?"=w342:bool)  [unwired: 3 in, 4 out]
          }
          frame True {
            n58 = for "For循环" {
              N: w348 -> [_]
              tunnel: w355 -> [w359]
              tunnel: [w364] -> w354
              tunnel: w353 -> [w361]
              tunnel: [w362] -> w352
              tunnel: w351 -> [_]
              tunnel: w349 -> [_]
              tunnel: w350 -> [_]
              tunnel: w347 -> [_]
              stop <- w363 stop-if-true
              n59 = Unbundle By Name(w361) -> ("TestResult"=w360:refnum<vi>)
              n60 = call "BootTimeTest.vi"("error in"=w359, "TestResult"=w360) -> ("error out"=w356:errorcluster, "BootTime"=w358:string)  [unwired: 8 in]
              n61 = call "TableHandle.vi"("All"=w361, "error in (no error)"=w356, "字符串数值"=TRUE, "DataIn"=w358) -> ("error out"=w364:errorcluster, "Stop?"=w362:bool, "StopForLoop"=w363:bool)  [unwired: 3 in, 2 out]
            }
          }
        }
      }
      frame "CANTest" {
        n62 = case shown="真" w377 {
          tunnel: w380 -> [w384 w395]
          tunnel: w379 -> [w385 w397]
          tunnel: [w386 w396] -> w378
          tunnel: [w383 w394] -> w376
          tunnel: w375 -> [_ w387]
          tunnel: w374 -> [_ w388]
          tunnel: w373 -> [_ w393]
          tunnel: w372 -> [_ w392]
          tunnel: w369 -> [_ w391]
          tunnel: [w381 w390] -> w368
          tunnel: w367 -> [w381 w389]
          frame False {
            n63 = call "TableHandle.vi"("All"=w384, "error in (no error)"=w385, "DataIn"=TRUE) -> ("error out"=w386:errorcluster, "Stop?"=w383:bool)  [unwired: 3 in, 4 out]
          }
          frame True {
            n64 = for "For循环" {
              N: w392 -> [_]
              tunnel: w397 -> [w411]
              tunnel: [w423] -> w396
              tunnel: w395 -> [w420]
              tunnel: [w421] -> w394
              tunnel: w393 -> [w412]
              tunnel: w388 -> [w403]
              tunnel: w391 -> [w419]
              shift-right: [w417] -> w390
              shift-left: w389 -> [w418]
              tunnel: w387 -> [_]
              stop <- w422 stop-if-true
              w398 = "\r\n"
              n65 = case shown="\"Slot1\", 默认" Slot."Slot1" ("Slot") {
                tunnel: [u32 0 ("CANChannel") u32 1 ("CANChannel")] -> w408
                frame "Slot1", Default {
                }
                frame "Slot2" {
                }
              }
              n66 = call "WaitTimes.vi"("WaitTimes"=u32 1000, "error in (no error)"=w411) -> ("error out"=w409:errorcluster)  [unwired: 9 in]
              n67 = Match Pattern(string=w403, regular expression=";") -> (before substring=w405:string, after substring=w401:string)  [unwired: 1 in, 2 out]
              n68 = call "CANTEST.vi"("Data Input(Hex)"=w412, "错误输入"=w409, "ID(Hex 高位有效)"=w403, "CANChannel"=w408) -> ("错误输出"=w407:errorcluster, "帧数据"=w399:string)  [unwired: 5 in, 1 out]
              n69 = Concatenate Strings(w418, "CAN发送:" ("字符串"), " ID:" ("字符串"), w405, " DATA:" ("字符串"), w412, w398, "接收ID:" ("字符串"), w401, " 接收数据:" ("字符串"), w399, w398) -> (w417:string)
              n70 = String Length(string=w417) -> (length=w416:i32)
              n71 = property class="Str"(reference=w419, "Text.Text"=w417, "Text.Scroll Position"=w416) -> ()  [unwired: 1 in, 2 out]
              n72 = call "TableHandle.vi"("All"=w420, "error in (no error)"=w407, "DataIn"=w399) -> ("error out"=w423:errorcluster, "Stop?"=w421:bool, "StopForLoop"=w422:bool)  [unwired: 4 in, 2 out]
            }
          }
        }
      }
      frame "CMD" {
        n73 = case shown="真" w441 {
          tunnel: w444 -> [w448 w464]
          tunnel: w443 -> [w449 w466]
          tunnel: [w450 w465] -> w442
          tunnel: [w447 w463] -> w440
          tunnel: w439 -> [_ w456]
          tunnel: w438 -> [_ w457]
          tunnel: w437 -> [_ w462]
          tunnel: w436 -> [_ w461]
          tunnel: w433 -> [_ w460]
          tunnel: [w445 w459] -> w432
          tunnel: w431 -> [w445 w458]
          tunnel: [w445 w455] -> w429
          tunnel: w428 -> [_ w454]
          tunnel: w427 -> [_ w453]
          tunnel: w426 -> [_ w452]
          frame False {
            n74 = call "TableHandle.vi"("All"=w448, "error in (no error)"=w449, "DataIn"=TRUE) -> ("error out"=w450:errorcluster, "Stop?"=w447:bool)  [unwired: 3 in, 4 out]
          }
          frame True {
            n75 = property class="Ring (严格)"(reference=w452) -> ("RingText.Text"=w451:string)  [unwired: 1 in, 2 out]
            n76 = for "For循环" {
              N: w461 -> [_]
              tunnel: w466 -> [w479]
              tunnel: [w492] -> w465
              tunnel: w464 -> [w489]
              tunnel: [w490] -> w463
              tunnel: w462 -> [w487]
              tunnel: w457 -> [w467]
              tunnel: w460 -> [w485]
              shift-right: [w483] -> w459
              shift-left: w458 -> [w484]
              tunnel: w456 -> [w469]
              tunnel: [w467] -> w455
              tunnel: w454 -> [w473]
              tunnel: w453 -> [w471]
              tunnel: w451 -> [w468]
              i -> [w480]
              stop <- w491 stop-if-true
              n77 = Decimal String To Number(string=w487, default (0L)=u32 0 ("默认(0 I32)")) -> (number=w477:u32)  [unwired: 1 in, 1 out]
              n78 = property class="Str"(reference=w471) -> ("Value"=w470:string)  [unwired: 1 in, 2 out]
              n79 = case shown="\"Slot2\"" w469 {
                tunnel: [w499 w500] -> w476
                frame "Slot1", Default {
                  n80 = global read "GlobalValue.vi" "Slot1COM"() -> (w499:refnum<visa-resource-name>)
                }
                frame "Slot2" {
                  n81 = global read "GlobalValue.vi" "Slot2COM"() -> (w500:refnum<visa-resource-name>)
                }
              }
              n82 = case shown="1, 默认" w480 {
                tunnel: w479 -> [w501 w504]
                tunnel: [w501 w503] -> w478
                tunnel: w477 -> [_ w502]
                frame 0 {
                }
                frame 1, Default {
                  n83 = call "WaitTimes.vi"("WaitTimes"=w502, "error in (no error)"=w504) -> ("error out"=w503:errorcluster)  [unwired: 9 in]
                }
              }
              n84 = call "CommunicationTool.vi"("VISA资源名称"=w476, "SN"=w470, "ModelNumber"=w468, "通信协议名称"=w467, "Slot"=w469, "DelayTime"=w477, "error in"=w478, "Debug"=FALSE) -> ("字符串数值"=w474:bool, "CMD"=w475:string, "data"=w472:string, "error out"=w488:errorcluster)  [unwired: 2 in, 2 out]
              n85 = Concatenate Strings(w484, w475) -> (w483:string)
              n86 = String Length(string=w483) -> (length=w482:i32)
              n87 = case shown="\"查询CCID\"" w467 {
                tunnel: w473 -> [_ w494 _]
                tunnel: w472 -> [_ w493 w495]
                tunnel: w469 -> [_ _ w496]
                frame "假", Default {
                }
                frame "查询版本", "查询版本(长丰)" {
                  n88 = property class="Str"(reference=w494, "Value"=w493) -> ()  [unwired: 1 in, 2 out]
                }
                frame "查询CCID" {
                  n89 = case shown="\"Slot2\"" w496 {
                    tunnel: w495 -> [w497 w498]
                    frame "Slot1", Default {
                      n90 = global write "GlobalValue.vi" "Slot1CCID"(w497) -> ()
                    }
                    frame "Slot2" {
                      n91 = global write "GlobalValue.vi" "Slot2CCID"(w498) -> ()
                    }
                  }
                }
              }
              n92 = property class="Str"(reference=w485, "Text.Text"=w483, "Text.Scroll Position"=w482) -> ()  [unwired: 1 in, 2 out]
              n93 = call "TableHandle.vi"("All"=w489, "error in (no error)"=w488, "字符串数值"=w474, "DataIn"=w472) -> ("error out"=w492:errorcluster, "Stop?"=w490:bool, "StopForLoop"=w491:bool)  [unwired: 3 in, 2 out]
            }
          }
        }
      }
      frame "CMD_360" {
        n94 = case shown="真" w521 {
          tunnel: w524 -> [w528 w545]
          tunnel: w523 -> [w529 w547]
          tunnel: [w530 w546] -> w522
          tunnel: [w527 w544] -> w520
          tunnel: w519 -> [_ w537]
          tunnel: w518 -> [_ w538]
          tunnel: w517 -> [_ w543]
          tunnel: w516 -> [_ w542]
          tunnel: w513 -> [_ w541]
          tunnel: [w525 w540] -> w512
          tunnel: w511 -> [w525 w539]
          tunnel: [w525 w536] -> w509
          tunnel: w508 -> [_ w535]
          tunnel: w507 -> [_ w534]
          tunnel: w506 -> [_ w533]
          tunnel: w505 -> [_ w531]
          frame False {
            n95 = call "TableHandle.vi"("All"=w528, "error in (no error)"=w529, "DataIn"=TRUE) -> ("error out"=w530:errorcluster, "Stop?"=w527:bool)  [unwired: 3 in, 4 out]
          }
          frame True {
            n96 = property class="Ring (严格)"(reference=w533) -> ("RingText.Text"=w532:string)  [unwired: 1 in, 2 out]
            n97 = for "For循环" {
              N: w542 -> [_]
              tunnel: w547 -> [w566]
              tunnel: [w578] -> w546
              tunnel: w545 -> [w575]
              tunnel: [w576] -> w544
              tunnel: w543 -> [w554]
              tunnel: w538 -> [w559]
              tunnel: w541 -> [w572]
              shift-right: [w570] -> w540
              shift-left: w539 -> [w571]
              tunnel: w537 -> [_]
              tunnel: [w559] -> w536
              tunnel: w535 -> [_]
              tunnel: w534 -> [w561]
              tunnel: w532 -> [_]
              tunnel: w531 -> [w557]
              i -> [w567]
              stop <- w577 stop-if-true
              n98 = Match Pattern(string=w554, regular expression=";" ("正则表达式")) -> (before substring=w552:string, after substring=w550:string)  [unwired: 1 in, 2 out]
              n99 = property class="Str"(reference=w561) -> ("Value"=w560:string)  [unwired: 1 in, 2 out]
              n100 = Decimal String To Number(string=w552, default (0L)=u32 0 ("默认(0 I32)")) -> (number=w564:u32)  [unwired: 1 in, 1 out]
              n101 = Decimal String To Number(string=w550, default (0L)=u32 0 ("默认(0 I32)")) -> (number=w549:u32)  [unwired: 1 in, 1 out]
              n102 = Equal To 0?(x=w549) -> (x = 0?=w548:bool)
              n103 = case shown="1, 默认" w567 {
                tunnel: w566 -> [w637 w640]
                tunnel: [w637 w639] -> w565
                tunnel: w564 -> [_ w638]
                frame 0 {
                }
                frame 1, Default {
                  n104 = call "WaitTimes.vi"("WaitTimes"=w638, "error in (no error)"=w640) -> ("error out"=w639:errorcluster)  [unwired: 9 in]
                }
              }
              n105 = case shown="\"Slot1\", 默认" Slot."Slot1" ("Slot") {
                tunnel: [w635 w636] -> w563
                frame "Slot1", Default {
                  n106 = global read "GlobalValue.vi" "Slot1COM"() -> (w635:refnum<visa-resource-name>)
                }
                frame "Slot2" {
                  n107 = global read "GlobalValue.vi" "Slot2COM"() -> (w636:refnum<visa-resource-name>)
                }
              }
              n108 = call "ComTool_360.vi"("Com"=w563, "SN"=w560, "通信协议名称"=w559, "DelayTime"=w564, "F0?"=w548, "error in"=w565, "Debug"=FALSE) -> ("Data"=w556:string, "CMD"=w562:string, "error out"=w574:errorcluster)  [unwired: 4 in, 2 out]
              n109 = case shown="\"3D后视视图\"" w557 {
                selector: w557 -> [_ w584 w595 w606 w617 w628]
                tunnel: w556 -> [w579 w581 w592 w603 w614 w625]
                tunnel: [w579 w583 w594 w605 w616 w627] -> w555
                frame "假", Default {
                }
                frame "2D前视视图" {
                  n110 = Equal?(x=w581, y="01") -> (x = y?=w582:bool)
                  n111 = case shown="真" w582 {
                    tunnel: w584 -> [_ w590]
                    tunnel: [w585 w589] -> w583
                    tunnel: w581 -> [w585 w587]
                    frame False {
                    }
                    frame True {
                      n112 = call "BulletFrame.vi"("StrIn"=w590) -> ("结果"=w588:bool)  [unwired: 1 in, 1 out]
                      n113 = Select(t=w587, s=w588, f="00") -> (s? t:f=w589:string)
                    }
                  }
                }
                frame "2D后视视图" {
                  n114 = Equal?(x=w592, y="02") -> (x = y?=w593:bool)
                  n115 = case shown="真" w593 {
                    tunnel: w595 -> [_ w601]
                    tunnel: [w596 w600] -> w594
                    tunnel: w592 -> [w596 w598]
                    frame False {
                    }
                    frame True {
                      n116 = call "BulletFrame.vi"("StrIn"=w601) -> ("结果"=w599:bool)  [unwired: 1 in, 1 out]
                      n117 = Select(t=w598, s=w599, f="00") -> (s? t:f=w600:string)
                    }
                  }
                }
                frame "2D左视视图" {
                  n118 = Equal?(x=w603, y="03") -> (x = y?=w604:bool)
                  n119 = case shown="真" w604 {
                    tunnel: w606 -> [_ w612]
                    tunnel: [w607 w611] -> w605
                    tunnel: w603 -> [w607 w609]
                    frame False {
                    }
                    frame True {
                      n120 = call "BulletFrame.vi"("StrIn"=w612) -> ("结果"=w610:bool)  [unwired: 1 in, 1 out]
                      n121 = Select(t=w609, s=w610, f="00") -> (s? t:f=w611:string)
                    }
                  }
                }
                frame "2D右视视图" {
                  n122 = Equal?(x=w614, y="04") -> (x = y?=w615:bool)
                  n123 = case shown="真" w615 {
                    tunnel: w617 -> [_ w623]
                    tunnel: [w618 w622] -> w616
                    tunnel: w614 -> [w618 w620]
                    frame False {
                    }
                    frame True {
                      n124 = call "BulletFrame.vi"("StrIn"=w623) -> ("结果"=w621:bool)  [unwired: 1 in, 1 out]
                      n125 = Select(t=w620, s=w621, f="00") -> (s? t:f=w622:string)
                    }
                  }
                }
                frame "3D后视视图" {
                  n126 = Equal?(x=w625, y="08") -> (x = y?=w626:bool)
                  n127 = case shown="真" w626 {
                    tunnel: w628 -> [_ w634]
                    tunnel: [w629 w633] -> w627
                    tunnel: w625 -> [w629 w631]
                    frame False {
                    }
                    frame True {
                      n128 = call "BulletFrame.vi"("StrIn"=w634) -> ("结果"=w632:bool)  [unwired: 1 in, 1 out]
                      n129 = Select(t=w631, s=w632, f="00") -> (s? t:f=w633:string)
                    }
                  }
                }
              }
              n130 = Concatenate Strings(w571, w562) -> (w570:string)
              n131 = String Length(string=w570) -> (length=w569:i32)
              n132 = property class="Str"(reference=w572, "Text.Text"=w570, "Text.Scroll Position"=w569) -> ()  [unwired: 1 in, 2 out]
              n133 = call "TableHandle.vi"("All"=w575, "error in (no error)"=w574, "DataIn"=w555) -> ("error out"=w578:errorcluster, "Stop?"=w576:bool, "StopForLoop"=w577:bool)  [unwired: 4 in, 2 out]
            }
          }
        }
      }
      frame "CheckSN" {
        n134 = case shown="真" w653 {
          tunnel: w656 -> [w660 w670]
          tunnel: w655 -> [w661 w672]
          tunnel: [w662 w671] -> w654
          tunnel: [w659 w669] -> w652
          tunnel: w651 -> [_ w668]
          tunnel: w650 -> [_ w667]
          tunnel: w649 -> [_ w666]
          tunnel: w648 -> [_ w665]
          tunnel: w647 -> [w657 w664]
          tunnel: [w657 w664] -> w646
          tunnel: w641 -> [_ w663]
          frame False {
            n135 = call "TableHandle.vi"("All"=w660, "error in (no error)"=w661, "DataIn"=TRUE) -> ("error out"=w662:errorcluster, "Stop?"=w659:bool)  [unwired: 3 in, 4 out]
          }
          frame True {
            n136 = for "For循环" {
              N: w665 -> [_]
              tunnel: w672 -> [w676]
              tunnel: [w682] -> w671
              tunnel: w670 -> [w679]
              tunnel: [w680] -> w669
              tunnel: w668 -> [w678]
              tunnel: w666 -> [_]
              tunnel: w667 -> [_]
              tunnel: w664 -> [_]
              tunnel: w663 -> [w675]
              stop <- w681 stop-if-true
              n137 = property class="Str"(reference=w675) -> ("Value"=w674:string)  [unwired: 1 in, 2 out]
              n138 = call "CheckSN.vi"("Slot"=w678, "error out"=w676, "SN"=w674) -> ("错误输出"=w677:errorcluster, "比对结果"=w673:bool)  [unwired: 7 in]
              n139 = global write "GlobalValue.vi" "SN Result"(w673) -> ()
              n140 = call "TableHandle.vi"("All"=w679, "error in (no error)"=w677, "DataIn"=w673) -> ("error out"=w682:errorcluster, "Stop?"=w680:bool, "StopForLoop"=w681:bool)  [unwired: 4 in, 2 out]
            }
          }
        }
      }
      frame "DIAction" {
        n141 = case shown="真" w693 {
          tunnel: w696 -> [w699 w707]
          tunnel: w695 -> [w700 w709]
          tunnel: [w701 w708] -> w694
          tunnel: [w698 w706] -> w692
          tunnel: w691 -> [_ w705]
          tunnel: w690 -> [_ w704]
          tunnel: w689 -> [_ w703]
          tunnel: w688 -> [_ w702]
          frame False {
            n142 = call "TableHandle.vi"("All"=w699, "error in (no error)"=w700, "DataIn"=TRUE) -> ("error out"=w701:errorcluster, "Stop?"=w698:bool)  [unwired: 3 in, 4 out]
          }
          frame True {
            n143 = for "For循环" {
              N: w702 -> [_]
              tunnel: w709 -> [w714]
              tunnel: [w718] -> w708
              tunnel: w707 -> [w715]
              tunnel: [w716] -> w706
              tunnel: w705 -> [w710]
              tunnel: w703 -> [_]
              tunnel: w704 -> [w712]
              stop <- w717 stop-if-true
              n144 = call "DIAction.vi"("Slot"=w710, "error in"=w714, "CH"=w712) -> ("error out"=w713:errorcluster, "Status"=w711:bool)  [unwired: 7 in]
              n145 = call "TableHandle.vi"("All"=w715, "error in (no error)"=w713, "DataIn"=w711) -> ("error out"=w718:errorcluster, "Stop?"=w716:bool, "StopForLoop"=w717:bool)  [unwired: 4 in, 2 out]
            }
          }
        }
      }
      frame "DOAction" {
        n146 = case shown="真" w729 {
          tunnel: w732 -> [w735 w743]
          tunnel: w731 -> [w736 w745]
          tunnel: [w737 w744] -> w730
          tunnel: [w734 w742] -> w728
          tunnel: w727 -> [_ w741]
          tunnel: w726 -> [_ w740]
          tunnel: w725 -> [_ w739]
          tunnel: w724 -> [_ w738]
          frame False {
            n147 = call "TableHandle.vi"("All"=w735, "error in (no error)"=w736, "DataIn"=TRUE) -> ("error out"=w737:errorcluster, "Stop?"=w734:bool)  [unwired: 3 in, 4 out]
          }
          frame True {
            n148 = for "For循环" {
              N: w738 -> [_]
              tunnel: w745 -> [w751]
              tunnel: [w755] -> w744
              tunnel: w743 -> [w752]
              tunnel: [w753] -> w742
              tunnel: w741 -> [w746]
              tunnel: w739 -> [w748]
              tunnel: w740 -> [w749]
              stop <- w754 stop-if-true
              n149 = call "DOAction.vi"("Slot"=w746, "error in"=w751, "State"=w748, "CH"=w749) -> ("error out"=w750:errorcluster)  [unwired: 7 in]
              n150 = call "TableHandle.vi"("All"=w752, "error in (no error)"=w750, "DataIn"="Done") -> ("error out"=w755:errorcluster, "Stop?"=w753:bool, "StopForLoop"=w754:bool)  [unwired: 4 in, 2 out]
            }
          }
        }
      }
      frame "Delay" {
        n151 = case shown="真" w766 {
          tunnel: w769 -> [w772 w780]
          tunnel: w768 -> [w773 w782]
          tunnel: [w774 w781] -> w767
          tunnel: [w771 w779] -> w765
          tunnel: w764 -> [_ w778]
          tunnel: w763 -> [_ w777]
          tunnel: w762 -> [_ w776]
          tunnel: w761 -> [_ w775]
          frame False {
            n152 = call "TableHandle.vi"("All"=w772, "error in (no error)"=w773, "DataIn"=TRUE) -> ("error out"=w774:errorcluster, "Stop?"=w771:bool)  [unwired: 3 in, 4 out]
          }
          frame True {
            n153 = for "For循环" {
              N: w775 -> [_]
              tunnel: w782 -> [w790]
              tunnel: [w794] -> w781
              tunnel: w780 -> [w791]
              tunnel: [w792] -> w779
              tunnel: w778 -> [_]
              tunnel: w776 -> [w786]
              tunnel: w777 -> [_]
              stop <- w793 stop-if-true
              n154 = Fract/Exp String To Number(string=w786) -> (number=w785:dbl)  [unwired: 3 in, 1 out]
              n155 = Multiply(x=w785, y=1000.0) -> (x*y=w784:dbl)
              n156 = To Unsigned Long Integer(number=w784) -> (unsigned 32bit integer=w783:u32)
              n157 = call "WaitTimes.vi"("WaitTimes"=w783, "error in (no error)"=w790) -> ("error out"=w789:errorcluster)  [unwired: 9 in]
              n158 = call "TableHandle.vi"("All"=w791, "error in (no error)"=w789, "DataIn"="Done") -> ("error out"=w794:errorcluster, "Stop?"=w792:bool, "StopForLoop"=w793:bool)  [unwired: 4 in, 2 out]
            }
          }
        }
      }
      frame "Frequency" {
        n159 = case shown="真" w806 {
          tunnel: w809 -> [w813 w822]
          tunnel: w808 -> [w814 w824]
          tunnel: [w815 w823] -> w807
          tunnel: [w812 w821] -> w805
          tunnel: w804 -> [_ w820]
          tunnel: w803 -> [_ w819]
          tunnel: w802 -> [_ w818]
          tunnel: w801 -> [_ w817]
          tunnel: w800 -> [w810 w816]
          tunnel: [w810 w816] -> w799
          frame False {
            n160 = call "TableHandle.vi"("All"=w813, "error in (no error)"=w814, "DataIn"=TRUE) -> ("error out"=w815:errorcluster, "Stop?"=w812:bool)  [unwired: 3 in, 4 out]
          }
          frame True {
            n161 = for "For循环" {
              N: w817 -> [_]
              tunnel: w824 -> [w828]
              tunnel: [w832] -> w823
              tunnel: w822 -> [w829]
              tunnel: [w830] -> w821
              tunnel: w820 -> [_]
              tunnel: w818 -> [_]
              tunnel: w819 -> [_]
              tunnel: w816 -> [w826]
              stop <- w831 stop-if-true
              n162 = call-poly <vilib>:"Extract Single Tone Information.vi"("error in (no error)"=w828, "time signal in"=w826) -> ("error out"=w827:errorcluster, "detected frequency"=w825:dbl)  [unwired: 4 in, 4 out]
              n163 = call "TableHandle.vi"("All"=w829, "error in (no error)"=w827, "DataIn"=w825) -> ("error out"=w832:errorcluster, "Stop?"=w830:bool, "StopForLoop"=w831:bool)  [unwired: 4 in, 2 out]
            }
          }
        }
      }
      frame "MeaCurrent" {
        n164 = case shown="真" w843 {
          tunnel: w846 -> [w849 w858]
          tunnel: w845 -> [w850 w860]
          tunnel: [w851 w859] -> w844
          tunnel: [w848 w857] -> w842
          tunnel: w841 -> [_ w856]
          tunnel: w840 -> [_ w855]
          tunnel: w839 -> [_ w854]
          tunnel: w838 -> [_ w853]
          tunnel: w833 -> [_ w852]
          frame False {
            n165 = call "TableHandle.vi"("All"=w849, "error in (no error)"=w850, "DataIn"=TRUE) -> ("error out"=w851:errorcluster, "Stop?"=w848:bool)  [unwired: 3 in, 4 out]
          }
          frame True {
            n166 = for "For循环" {
              N: w853 -> [_]
              tunnel: w860 -> [w870]
              tunnel: [w877] -> w859
              tunnel: w858 -> [w874]
              tunnel: [w875] -> w857
              tunnel: w856 -> [w871]
              tunnel: w854 -> [w873]
              tunnel: w855 -> [w872]
              tunnel: w852 -> [w867]
              i -> [w866]
              stop <- w876 stop-if-true
              w862 = 3
              n167 = case shown="\"Slot1\", 默认" w871 {
                tunnel: [w892 w893] -> w868
                frame "Slot1", Default {
                  n168 = global read "GlobalValue.vi" "Slot1COM"() -> (w892:refnum<visa-resource-name>)
                }
                frame "Slot2" {
                  n169 = global read "GlobalValue.vi" "Slot2COM"() -> (w893:refnum<visa-resource-name>)
                }
              }
              n170 = case shown="1, 默认" w866 {
                tunnel: w870 -> [w885 w890]
                tunnel: [w885 w889] -> w869
                tunnel: w868 -> [_ w888]
                tunnel: w867 -> [_ w887]
                frame 0 {
                }
                frame 1, Default {
                  n171 = call "CommunicationTool.vi"("VISA资源名称"=w888, "通信协议名称"=w887, "DelayTime"=u32 1000, "error in"=w890, "Debug"=FALSE) -> ("error out"=w889:errorcluster)  [unwired: 5 in, 5 out]
                }
              }
              n172 = for {
                N: w862 -> [_]
                tunnel: w873 -> [w884]
                tunnel: w872 -> [w883]
                tunnel: w871 -> [w882]
                tunnel: w869 -> [w881]
                tunnel: [w878] -> w864 mode=indexing
                shift-right: [w880] -> w865
                shift-left: _ -> [_]
                n173 = Build Array(w883) -> (w879:string[])
                n174 = call "AIs-Freq.vi"("Slot"=w882, "error in"=w881, "Mode"=w884, "CHs"=w879) -> ("error out"=w880:errorcluster, "RMS value"=w878:dbl)  [unwired: 5 in, 1 out]
              }
              n175 = Add Array Elements(numeric array=w864) -> (sum=w863:dbl)
              n176 = Divide(x=w863, y=w862) -> (x/y=w861:dbl)
              n177 = call "TableHandle.vi"("All"=w874, "error in (no error)"=w865, "DataIn"=w861) -> ("error out"=w877:errorcluster, "Stop?"=w875:bool, "StopForLoop"=w876:bool)  [unwired: 4 in, 2 out]
            }
          }
        }
      }
      frame "RMS" {
        n178 = case shown="真" w906 {
          tunnel: w909 -> [w913 w923]
          tunnel: w908 -> [w914 w925]
          tunnel: [w915 w924] -> w907
          tunnel: [w912 w922] -> w905
          tunnel: w904 -> [_ w921]
          tunnel: w903 -> [_ w920]
          tunnel: w902 -> [_ w919]
          tunnel: w901 -> [_ w918]
          tunnel: w900 -> [w910 w917]
          tunnel: [w910 w917] -> w899
          tunnel: w896 -> [_ w916]
          frame False {
            n179 = call "TableHandle.vi"("All"=w913, "error in (no error)"=w914, "DataIn"=TRUE) -> ("error out"=w915:errorcluster, "Stop?"=w912:bool)  [unwired: 3 in, 4 out]
          }
          frame True {
            n180 = for "For循环" {
              N: w918 -> [_]
              tunnel: w925 -> [w932]
              tunnel: [w938] -> w924
              tunnel: w923 -> [w935]
              tunnel: [w936] -> w922
              tunnel: w921 -> [w926]
              tunnel: w919 -> [_]
              tunnel: w920 -> [_]
              tunnel: w917 -> [w929]
              tunnel: w916 -> [w928]
              i -> [w927]
              stop <- w937 stop-if-true
              n181 = case shown="1, 默认" w927 {
                tunnel: w932 -> [w940 w951]
                tunnel: [w940 w950] -> w931
                tunnel: w928 -> [_ w949]
                tunnel: w926 -> [_ w945]
                tunnel: [w939 w946] -> w930
                tunnel: w929 -> [w939 _]
                frame 0 {
                }
                frame 1, Default {
                  n182 = call "GlobalVariable.vi"("Name"="CH", "Slot"=w945) -> ("String"=w944:string)  [unwired: 10 in, 3 out]
                  n183 = call "GlobalVariable.vi"("Name"="Para", "Slot"=w945) -> ("String"=w941:string)  [unwired: 10 in, 3 out]
                  n184 = Build Array(w944) -> (w948:string[])
                  n185 = call "AIs-Freq.vi"("Slot"=w945, "error in"=w951, "Mode"=w941, "CHs"=w948) -> ("error out"=w950:errorcluster, "波形图"=w947:waveform(dbl)[])  [unwired: 5 in, 1 out]
                  n186 = property class="WFGraph (严格)"(reference=w949, "Value"=w947, "XScale.Minimum"=0.0 ("X标尺.范围:最小值"), "XScale.Maximum"=0.01 ("X标尺.范围:最大值")) -> ()  [unwired: 1 in, 2 out]
                  n187 = Index Array(array=w947) -> (element=w946:waveform(dbl))  [unwired: 1 in]
                }
              }
              n188 = call-poly <vilib>:"Basic Averaged DC-RMS.vi"("error in (no error)"=w931, "signal in"=w930) -> ("error out"=w934:errorcluster, "RMS value"=w933:dbl)  [unwired: 6 in, 2 out]
              n189 = call "TableHandle.vi"("All"=w935, "error in (no error)"=w934, "DataIn"=w933) -> ("error out"=w938:errorcluster, "Stop?"=w936:bool, "StopForLoop"=w937:bool)  [unwired: 4 in, 2 out]
            }
          }
        }
      }
      frame "SNR" {
        n190 = case shown="真" w966 {
          tunnel: w969 -> [w973 w983]
          tunnel: w968 -> [w974 w985]
          tunnel: [w975 w984] -> w967
          tunnel: [w972 w982] -> w965
          tunnel: w964 -> [_ w981]
          tunnel: w963 -> [_ w980]
          tunnel: w962 -> [_ w979]
          tunnel: w961 -> [_ w978]
          tunnel: w960 -> [w970 w977]
          tunnel: [w970 w977] -> w959
          tunnel: w956 -> [_ w976]
          frame False {
            n191 = call "TableHandle.vi"("All"=w973, "error in (no error)"=w974, "DataIn"=TRUE) -> ("error out"=w975:errorcluster, "Stop?"=w972:bool)  [unwired: 3 in, 4 out]
          }
          frame True {
            n192 = for "For循环" {
              N: w978 -> [_]
              tunnel: w985 -> [w992]
              tunnel: [w998] -> w984
              tunnel: w983 -> [w995]
              tunnel: [w996] -> w982
              tunnel: w981 -> [w987]
              tunnel: w979 -> [_]
              tunnel: w980 -> [_]
              tunnel: w977 -> [w989]
              tunnel: w976 -> [w988]
              i -> [w986]
              stop <- w997 stop-if-true
              n193 = case shown="1, 默认" w986 {
                tunnel: w992 -> [w1010 w1021]
                tunnel: [w1010 w1020] -> w991
                tunnel: w988 -> [_ w1019]
                tunnel: w987 -> [_ w1011]
                tunnel: [w1009 w1017] -> w990
                tunnel: w989 -> [w1009 _]
                frame 0 {
                }
                frame 1, Default {
                  n194 = call "GlobalVariable.vi"("Name"="CH", "Slot"=w1011) -> ("String"=w1013:string)  [unwired: 10 in, 3 out]
                  n195 = call "GlobalVariable.vi"("Name"="Para", "Slot"=w1011) -> ("String"=w1012:string)  [unwired: 10 in, 3 out]
                  n196 = Build Array(w1013) -> (w1018:string[])
                  n197 = call "AIs-Freq.vi"("Slot"=w1011, "error in"=w1021, "Mode"=w1012, "CHs"=w1018) -> ("error out"=w1020:errorcluster, "波形图"=w1016:waveform(dbl)[])  [unwired: 5 in, 1 out]
                  n198 = property class="WFGraph (严格)"(reference=w1019, "Value"=w1016, "XScale.Minimum"=0.0 ("X标尺.范围:最小值"), "XScale.Maximum"=0.01 ("X标尺.范围:最大值")) -> ()  [unwired: 1 in, 2 out]
                  n199 = Index Array(array=w1016) -> (element=w1017:waveform(dbl))  [unwired: 1 in]
                }
              }
              n200 = disable-structure shown="启用" {
                disable-tunnel: [w1004 w1008] -> w994
                disable-tunnel: [w1002 w1006] -> w993
                disable-tunnel: w991 -> [w1000 w1008]
                disable-tunnel: w990 -> [w999 w1007]
                frame Disabled {
                  n201 = call-poly <vilib>:"Basic Averaged DC-RMS.vi"("reset"=TRUE, "error in (no error)"=w1000, "signal in"=w999) -> ("error out"=w1004:errorcluster, "RMS value"=w1005:dbl)  [unwired: 5 in, 2 out]
                  n202 = expression code="20*log(x)"(w1005) -> (w1003:dbl)
                  n203 = Absolute Value(x=w1003) -> (abs(x)=w1002:dbl)
                }
                frame Enabled {
                  n204 = call-poly <vilib>:"SINAD Analyzer.vi"("signal in"=w1007) -> ("SINAD (dB)"=w1006:dbl)  [unwired: 5 in, 5 out]
                }
              }
              n205 = call "TableHandle.vi"("All"=w995, "error in (no error)"=w994, "DataIn"=w993) -> ("error out"=w998:errorcluster, "Stop?"=w996:bool, "StopForLoop"=w997:bool)  [unwired: 4 in, 2 out]
            }
          }
        }
      }
      frame "Signal" {
        n206 = case shown="真" w1034 {
          tunnel: w1037 -> [w1040 w1048]
          tunnel: w1036 -> [w1041 w1050]
          tunnel: [w1042 w1049] -> w1035
          tunnel: [w1039 w1047] -> w1033
          tunnel: w1032 -> [_ w1046]
          tunnel: w1031 -> [_ w1045]
          tunnel: w1030 -> [_ w1044]
          tunnel: w1029 -> [_ w1043]
          frame False {
            n207 = call "TableHandle.vi"("All"=w1040, "error in (no error)"=w1041, "DataIn"=TRUE) -> ("error out"=w1042:errorcluster, "Stop?"=w1039:bool)  [unwired: 3 in, 4 out]
          }
          frame True {
            n208 = for "For循环" {
              N: w1043 -> [_]
              tunnel: w1050 -> [w1056]
              tunnel: [w1060] -> w1049
              tunnel: w1048 -> [w1057]
              tunnel: [w1058] -> w1047
              tunnel: w1046 -> [w1051]
              tunnel: w1044 -> [w1053]
              tunnel: w1045 -> [w1054]
              stop <- w1059 stop-if-true
              n209 = call "DOFreq.vi"("Slot"=w1051, "error in"=w1056, "State"=w1053, "CH"=w1054) -> ("error out"=w1055:errorcluster)  [unwired: 7 in]
              n210 = call "TableHandle.vi"("All"=w1057, "error in (no error)"=w1055, "DataIn"="Done") -> ("error out"=w1060:errorcluster, "Stop?"=w1058:bool, "StopForLoop"=w1059:bool)  [unwired: 4 in, 2 out]
            }
          }
        }
      }
      frame "Static Current" {
        n211 = case shown="真" w1061 {
          tunnel: w1066 -> [w1077 w1085]
          tunnel: w1067 -> [w1078 w1087]
          tunnel: [w1079 w1086] -> w1063
          tunnel: [w1076 w1084] -> w1064
          tunnel: w1065 -> [_ w1083]
          tunnel: w1069 -> [_ w1082]
          tunnel: w1068 -> [_ w1081]
          tunnel: w1070 -> [_ w1080]
          frame False {
            n212 = call "TableHandle.vi"("All"=w1077, "error in (no error)"=w1078, "DataIn"=TRUE) -> ("error out"=w1079:errorcluster, "Stop?"=w1076:bool)  [unwired: 3 in, 4 out]
          }
          frame True {
            n213 = for "For循环" {
              N: w1080 -> [_]
              tunnel: w1087 -> [_]
              tunnel: [w1098] -> w1086
              tunnel: w1085 -> [w1095]
              tunnel: [w1096] -> w1084
              tunnel: w1083 -> [w1094]
              tunnel: w1081 -> [w1088]
              tunnel: w1082 -> [w1089]
              stop <- w1097 stop-if-true
              n214 = case shown="\"Slot1\", 默认" w1094 {
                tunnel: [w1109 w1110] -> w1093
                frame "Slot1", Default {
                  n215 = global read "GlobalValue.vi" "Slot1QCCOM"() -> (w1109:refnum<visa-resource-name>)
                }
                frame "Slot2" {
                  n216 = global read "GlobalValue.vi" "Slot2QCCOM"() -> (w1110:refnum<visa-resource-name>)
                }
              }
              n217 = case shown="\"Vol\", 默认" w1088 {
                tunnel: [w1099 w1100] -> w1092
                frame "Vol", Default {
                  w1099 = u16 0 items=["DCV", "ACV", "DCI", "ACI", "OHM", "RST", "CAP", "FRQ", "AUTO"] ("测试类型")
                }
                frame "Curr" {
                  w1100 = u16 2 items=["DCV", "ACV", "DCI", "ACI", "OHM", "RST", "CAP", "FRQ", "AUTO"] ("测试类型")
                }
              }
              n218 = case shown="\"UT805A\"" w1089 {
                tunnel: w1093 -> [w1104 w1108]
                tunnel: w1092 -> [w1103 w1107]
                tunnel: [w1102 w1106] -> w1091
                tunnel: [w1101 w1105] -> w1090
                frame "GDM8341", Default {
                  n219 = call "Meacurrent8341.vi"("测试类型"=w1103, "VISA资源名称"=w1104) -> ("错误输出"=w1101:errorcluster, "数值"=w1102:dbl)  [unwired: 7 in, 1 out]
                }
                frame "UT805A" {
                  n220 = call "Meacurrent.vi"("测试类型"=w1107, "VISA资源名称"=w1108) -> ("错误输出"=w1105:errorcluster, "数值"=w1106:dbl)  [unwired: 8 in]
                }
              }
              "错误输出" <- w1090
              n221 = call "TableHandle.vi"("All"=w1095, "DataIn"=w1091) -> ("error out"=w1098:errorcluster, "Stop?"=w1096:bool, "StopForLoop"=w1097:bool)  [unwired: 5 in, 2 out]
            }
          }
        }
      }
      frame "StopTest" {
        # "此步骤不能删除"
      }
      frame "THD" {
        n222 = case shown="真" w1130 {
          tunnel: w1133 -> [w1137 w1147]
          tunnel: w1132 -> [w1138 w1149]
          tunnel: [w1139 w1148] -> w1131
          tunnel: [w1136 w1146] -> w1129
          tunnel: w1128 -> [_ w1145]
          tunnel: w1127 -> [_ w1144]
          tunnel: w1126 -> [_ w1143]
          tunnel: w1125 -> [_ w1142]
          tunnel: w1124 -> [w1134 w1141]
          tunnel: [w1134 w1141] -> w1123
          tunnel: w1120 -> [_ w1140]
          frame False {
            n223 = call "TableHandle.vi"("All"=w1137, "error in (no error)"=w1138, "DataIn"=TRUE) -> ("error out"=w1139:errorcluster, "Stop?"=w1136:bool)  [unwired: 3 in, 4 out]
          }
          frame True {
            n224 = for "For循环" {
              N: w1142 -> [_]
              tunnel: w1149 -> [w1156]
              tunnel: [w1163] -> w1148
              tunnel: w1147 -> [w1154]
              tunnel: [w1161] -> w1146
              tunnel: w1145 -> [w1152]
              tunnel: w1143 -> [_]
              tunnel: w1144 -> [_]
              tunnel: w1141 -> [w1150]
              tunnel: w1140 -> [w1153]
              i -> [w1157]
              stop <- w1162 stop-if-true
              n225 = case shown="1, 默认" w1157 {
                tunnel: w1156 -> [w1165 w1176]
                tunnel: [w1165 w1175] -> w1155
                tunnel: w1153 -> [_ w1174]
                tunnel: w1152 -> [_ w1170]
                tunnel: [w1164 w1171] -> w1151
                tunnel: w1150 -> [w1164 _]
                frame 0 {
                }
                frame 1, Default {
                  n226 = call "GlobalVariable.vi"("Name"="CH", "Slot"=w1170) -> ("String"=w1169:string)  [unwired: 10 in, 3 out]
                  n227 = call "GlobalVariable.vi"("Name"="Para", "Slot"=w1170) -> ("String"=w1168:string)  [unwired: 10 in, 3 out]
                  n228 = Build Array(w1169) -> (w1173:string[])
                  n229 = call "AIs-Freq.vi"("Slot"=w1170, "error in"=w1176, "Mode"=w1168, "CHs"=w1173) -> ("error out"=w1175:errorcluster, "波形图"=w1172:waveform(dbl)[])  [unwired: 5 in, 1 out]
                  n230 = property class="WFGraph (严格)"(reference=w1174, "Value"=w1172, "XScale.Minimum"=0.0 ("X标尺.范围:最小值"), "XScale.Maximum"=0.01 ("X标尺.范围:最大值")) -> ()  [unwired: 1 in, 2 out]
                  n231 = Index Array(array=w1172) -> (element=w1171:waveform(dbl))  [unwired: 1 in]
                }
              }
              n232 = call-poly <vilib>:"SVT THD+N.vi"("scaled signal [EU]"=w1151, "error in (no error)"=w1155, "desired units"=T5 {"THD+N units"=enum."%", "detected fundamental amplitude units"=enum."EU rms"}) -> ("THD+N"=w1158:dbl, "error out"=w1160:errorcluster)  [unwired: 11 in, 4 out]
              n233 = call "TableHandle.vi"("All"=w1154, "error in (no error)"=w1160, "DataIn"=w1158) -> ("error out"=w1163:errorcluster, "Stop?"=w1161:bool, "StopForLoop"=w1162:bool)  [unwired: 4 in, 2 out]
            }
          }
        }
      }
      frame "WDataToDB" {
        n234 = global read "GlobalValue.vi" "SN Result"() -> (w1181:bool)
        n235 = case shown="真" w1181 {
          tunnel: w1191 -> [_ w1208]
          tunnel: w1190 -> [_ w1202]
          tunnel: w1189 -> [_ w1207]
          tunnel: w1188 -> [_ w1206]
          tunnel: ["SN FAIL" ("ResultA") w1204] -> w1185
          tunnel: [w1198 w1205] -> w1183
          tunnel: w1182 -> [w1198 w1205]
          tunnel: [errorcluster {"status"=FALSE, "code"=0, "source"=""} ("错误输出") w1200] -> w1180
          frame False {
          }
          frame True {
            n236 = flat-sequence {
              tunnel: w1208 -> [w1215]
              tunnel: w1207 -> [w1214]
              tunnel: w1206 -> [w1213]
              tunnel: [w1212] -> w1204
              tunnel: w1202 -> [w1209]
              tunnel: [w1211] -> w1201
              tunnel: [w1210] -> w1200
              tunnel: [w1209] -> w1199
              frame #0 {
                n237 = xnode "错误下拉列表"() -> ("错误输出"=w1210:errorcluster)
                n238 = call "WriteDataToDB.vi"("通信协议名称"=w1215, "SN"=w1213, "产品型号"=w1214, "Slot"=w1209) -> ("ResultA"=w1212:string, "FSNA"=w1211:string)  [unwired: 6 in]
              }
            }
            n239 = call "ccidinfo-w.vi"("Data"=w1201, "Data Type"=CCID_info."DevID", "Slot"=w1199) -> ()  [unwired: 1 in]
          }
        }
        n240 = call "TableHandle.vi"("All"=w1183, "error in (no error)"=w1180, "字符串数值"=FALSE, "DataIn"=w1185) -> ("error out"=w1187:errorcluster, "Stop?"=w1186:bool)  [unwired: 3 in, 3 out]
      }
      frame "Wait" {
      }
      frame "幅度DB" {
        n241 = case shown="真" w1235 {
          tunnel: w1238 -> [w1242 w1251]
          tunnel: w1237 -> [w1243 w1253]
          tunnel: [w1244 w1252] -> w1236
          tunnel: [w1241 w1250] -> w1234
          tunnel: w1233 -> [_ w1249]
          tunnel: w1232 -> [_ w1248]
          tunnel: w1231 -> [_ w1247]
          tunnel: w1230 -> [_ w1246]
          tunnel: w1229 -> [w1239 w1245]
          tunnel: [w1239 w1245] -> w1228
          frame False {
            n242 = call "TableHandle.vi"("All"=w1242, "error in (no error)"=w1243, "DataIn"=TRUE) -> ("error out"=w1244:errorcluster, "Stop?"=w1241:bool)  [unwired: 3 in, 4 out]
          }
          frame True {
            n243 = for "For循环" {
              N: w1246 -> [_]
              tunnel: w1253 -> [w1257]
              tunnel: [w1262] -> w1252
              tunnel: w1251 -> [w1259]
              tunnel: [w1260] -> w1250
              tunnel: w1249 -> [_]
              tunnel: w1247 -> [_]
              tunnel: w1248 -> [_]
              tunnel: w1245 -> [w1258]
              stop <- w1261 stop-if-true
              n244 = call-poly <vilib>:"Basic Averaged DC-RMS.vi"("error in (no error)"=w1257, "signal in"=w1258) -> ("error out"=w1256:errorcluster, "RMS value"=w1255:dbl)  [unwired: 6 in, 2 out]
              n245 = expression code="20*log(x)"(w1255) -> (w1254:dbl)
              n246 = call "TableHandle.vi"("All"=w1259, "error in (no error)"=w1256, "DataIn"=w1254) -> ("error out"=w1262:errorcluster, "Stop?"=w1260:bool, "StopForLoop"=w1261:bool)  [unwired: 4 in, 2 out]
            }
          }
        }
      }
      frame "空", Default {
        # "此步骤不能删除"
        n247 = case shown="\"Slot4\"" w1266 {
          tunnel: ["Slot1 " ("字符串") "Slot2 " ("字符串") "Slot3 " ("字符串") "Slot4 " ("字符串")] -> w1265
          frame "Slot1", Default {
          }
          frame "Slot2" {
          }
          frame "Slot3" {
          }
          frame "Slot4" {
          }
        }
        n248 = Concatenate Strings(w1265, "Cann't find the \"" ("source"), w1271, "\" item." ("字符串")) -> (w1270:string)
        n249 = Bundle By Name(cluster=errorcluster {"status"=TRUE, "code"=5000, "source"=""} ("error in 1 (no error)"), "source"=w1270) -> (w1275:errorcluster)
      }
    }
  }
  "error out" <- w9
